vi "App - temperature sweep -- Pgg2.vi"() -> ()   [LabVIEW 2016]
uses:
  <vilib>/regexp/Match Regular Expression.xnode
  pair.ctl
  p9action control.ctl
  itc 503 box - control.ctl
  gas flow controller action.ctl
  ctl -- name dispatcher -- action.ctl
  countdown control.ctl
  NHMFL_Core/Libraries/Instruments/Temperature Controller/Controls/Set Point Aproach.ctl
  state.ctl
  save log.ctl
  resonant_ultrasound/Libraries/RUS/Controls/Sweep settings.ctl
  resonant_ultrasound/Libraries/RUS/Controls/Lock-in DAQ settings.ctl
  NHMFL_Core/Libraries/File/Controls/File formats.ctl
  NHMFL_Core/Libraries/File/Controls/Save data settings.ctl
  alarm clock control.ctl
  temperature indicator.ctl
  gas flow control - progress.ctl
  adaptive sweep UI controls.ctl
  next chunk -- algorithm.ctl
  Set Temperature PID - Control.ctl
  time in gamma mode control.ctl
  Sample_Temperature_Source_Control.ctl
  ITC Panel -- Hg.ctl
  gas flow controller control -- Pgg2.ctl
  resonant_ultrasound/Libraries/RUS/Controls/Lockin mode.ctl
  oxford ITC legacy-new - control.ctl
panel:
  in  "sweep folder path":path=path "C:/data/Ultrasound/birdcage/0_test"
  in  "Tab: everything":T1(tab) caption="Tab Control"
  in  "Tab: RUS controls":T2(tab)
  in  "RUS settings":enum32{"main", "save and staff"}(tab)
  in  "adaptive sweep settings":T3={"time gap (min) "=0.0, "Bypass error dialog"=TRUE, "range factor"=1.2, "min gamma(kHz)"=0.005, "max step(Hz)"=1500.0, "min step(Hz)"=0.001, "save freq units"=enum."kHz", "Zero signal?"=FALSE, "time in Gamma --OK"=FALSE, "scan mode"=enum."uniform", "power control mode "=enum."none", "time-in-gamma mode"=enum."uniform scan"}
  in  "Fast sweep settings":T6={"Update rate (Hz)"=200.0, "Start F, Hz"=2000000.0, "Stop F"=3000000.0, "Number of points"=5760, "Amplitude"=2.0, "Init&amplitude"=TRUE, "IF"=1000.0, "Time constant"=0.001} {"IF" format="%#_6p"; "Amplitude" min=0.0 max=2.5; "Number of points" format="%.0p"; "Stop F" format="%#_6p"; "Start F, Hz" format="%#_6p"; "Update rate (Hz)" format="%0.2f"}
  in  "Save data settings":T7={"Save data"=TRUE, "Data Root Path"=path "E:/Technique/RUS/Saphire/Saphire_piece1/1_test", "File Prefix"="291.30300K_2000_3000_2.00000V_0.00000T_Jul26-2016__14-58-15_", "File Format"=enum."BINARY", "Save column names"=FALSE, "File Comments"="\r\nColumns:Frequency\\tX\\tY\r\n    ITC Temp= 299.200000\r\n    LTC Temp= 0.000000\r\n          ITC_set=295.00000\r\n", "User/Prj"="<User Name/Project Description>"}
  in  "Lock-in DAQ settings":T9={"Lockin mode"=enum."Pitaya", "DAQmx Device"="", "SR Lockin"="GPIB0::10::INSTR", "Clock Multiplier"=64, "Low-pass filter"=enum."No filtering", "Ranges and couplings "=[{"Range"=2.5, "Coupling"=10106}], "Samples per read"=20, "Record IF"=FALSE, "Auto-phase"=FALSE, "RP IP Addres"="172.20.117.190"} {"Ranges and couplings"."Coupling" items=["default"=-1, "RSE"=10083, "NRSE"=10078, "Differential"=10106, "Pseudodifferential"=12529]}
  out "sweep time  (min)":dbl=1.05
  out "sweep time (sec)":i32=63
  out "kHz/second":dbl=31.746031746031747
  in  "RUS loop":bool
  in  "RUS zeroed":bool
  in  "read AH every # sec":dbl=1.7
  in  "plot":T11(ring)=enum."Capac vs Temp"
  out "temperature":dbl=198.969
  out "time(min)":dbl
  out "Capacitance":dbl=0.600435
  out "Loss":dbl=0.00206
  in  "save every # (min)":dbl=7.12
  in  "history length (min)":dbl=60.0
  in  "Sweep folder path":path=path "C:/data/RUS/Experiment/ProbeTest/cantilever/Hg1201-2-2/sweep1"
  in  "VISA - AH2500":refnum<visa-resource-name>="GPIB0::28::INSTR"
  in  "take cantilever reading":bool=TRUE
  out "Plot: capacitance":cluster{dbl[], dbl[]}[](graph)
  in  "plot lever  ?":bool
  in  "show plot pallets ?":bool
  in  "Tab: ITC controls":enum32{"display", "gas ", "progress"}(tab)
  in  "set Temperature target":T12(ring)=enum."set T -> ITC (oxford)"
  in  "Set Temperature PID":T13={"mode "=enum."bezier", "set temperature?"=FALSE, "Time(min)"=1492.1025, "Temperature(K)"=295.0, "OK?"=TRUE, "interval(sec)"=6.153}
  in  "ITC panel":T14={"in sweep"=FALSE, "start/stop sweep"=FALSE, "ITC state"="X0A1C2S01H1L0\r", "gas MANUAL"=TRUE, "gas AUTO"=FALSE, "local"=TRUE, "unlocked"=TRUE, "remote"=FALSE, "locked"=FALSE, "gas (%)"=0.0999, "heater AUTO"=FALSE, "heater MANUAL"=TRUE, "state indicator  (fake)"="NOT in sweep", "heater (V)"=0.0001, "Sweep"=FALSE}
  in  "itc box: set temperature to: value":dbl=295.0
  in  "set temperature to":bool
  in  "interaction with itc":T15(ring)
  in  "set heater to":bool
  in  "itc box: set heater to: value":dbl
  in  "itc box protocol selector":T16
  in  "gas flow controller":T17={"UP step (%)"=0.5, "ramp DOWN"=FALSE, "ramp UP"=FALSE, "idle"=TRUE, "UP time (min)"=20.0, "ramp step (%)"=0.1, "check (min)"=3.0, "DOWN step (%)"=0.5, "DOWN time (min)"=20.0, "to"=0.1, "last (min)"=1.6407999999999996, "below"=TRUE, "above"=FALSE, "Control Gas"=FALSE, "upper"=7.0, "lower"=3.0, "heater"=0.00010000000000000003, "in range"=FALSE, "gas, %"=0.0999, "ramp Up progress"={"(total # of ramp steps)"=5, "ramp time step (sec)"=240, "steps so far"=0, "state"=enum."normal"}, "ramp Down progress"={"(total # of ramp steps)"=5, "ramp time step (sec)"=240, "steps so far"=0, "state"=enum."normal"}, "state"=enum."normal", "set gas"=FALSE}
  out "ramp Down progress":T18={"(total # of ramp steps)"=5, "ramp time step (sec)"=240, "steps so far"=0, "state"=enum."normal"}
  out "ramp Up progress":T18={"(total # of ramp steps)"=5, "ramp time step (sec)"=240, "steps so far"=0, "state"=enum."normal"}
  in  "Tab: plots":enum32{"Plot:  gas/heater", "Plot: temperayre"}(tab)=enum."Plot: temperayre"
  out "Plot: heater/gas":cluster{dbl[], dbl[]}[](graph)
  out "Plot: temperature":cluster{dbl[], dbl[]}[](graph)=[{array[586 elements], [0.0, 0.0, 0.0, 0.0, 0.0, 0.0, 0.0, 0.0, 0.0, 0.0, 0.0, 0.0, 0.0, 0.0, 0.0, 0.0, 0.0, 0.0, 0.0, 0.0, 0.0, 0.0, 0.0, 0.0, 0.0, 0.0, 0.0, 0.0, 0.0, 0.0, 0.0, 0.0, 0.0, 0.0, 0.0, 0.0, 0.0, 0.0, 0.0, 0.0, 0.0, 0.0, 0.0, 0.0, 0.0, 0.0, 0.0, 0.0, 0.0, 0.0, 0.0, 0.0, 0.0, 0.0, 0.0, 0.0, 0.0, 0.0, 0.0, 0.0, 0.0, 0.0, 0.0, 0.0, 0.0, 0.0, 0.0, 0.0, 0.0, 0.0, 0.0, 0.0, 0.0, 0.0, 0.0, 0.0, 0.0, 0.0, 0.0, 0.0, 0.0, 0.0, 0.0, 0.0, 0.0, 0.0, 0.0, 0.0, 0.0, 0.0, 0.0, 0.0, 0.0, 0.0, 0.0, 0.0, 0.0, 0.0, 0.0, 0.0, 0.0, 0.0, 0.0, 0.0, 0.0, 0.0, 0.0, 0.0, 0.0, 0.0, 0.0, 0.0, 0.0, 0.0, 0.0, 0.0, 0.0, 0.0, 0.0, 0.0, 0.0, 0.0, 0.0, 0.0, 0.0, 0.0, 0.0, 0.0, 0.0, 0.0, 0.0, 0.0, 0.0, 0.0, 0.0, 0.0, 0.0, 0.0, 0.0, 0.0, 0.0, 0.0, 0.0, 0.0, 0.0, 0.0, 0.0, 0.0, 0.0, 0.0, 0.0, 0.0, 0.0, 0.0, 0.0, 0.0, 0.0, 0.0, 0.0, 0.0, 0.0, 0.0, 0.0, 0.0, 0.0, 0.0, 0.0, 0.0, 0.0, 0.0, 0.0, 0.0, 0.0, 0.0, 0.0, 0.0, 0.0, 0.0, 0.0, 0.0, 0.0, 0.0, 0.0, 0.0, 0.0, 0.0, 0.0, 0.0, 0.0, 0.0, 0.0, 0.0, 0.0, 0.0, 0.0, 0.0, 0.0, 0.0, 0.0, 0.0, 0.0, 0.0, 0.0, 0.0, 0.0, 0.0, 0.0, 0.0, 0.0, 0.0, 0.0, 0.0, 0.0, 0.0, 0.0, 0.0, 0.0, 0.0, 0.0, 0.0, 0.0, 0.0, 0.0, 0.0, 0.0, 0.0, 0.0, 0.0, 0.0, 0.0, 0.0, 0.0, 0.0, 0.0, 0.0, 0.0, 0.0, 0.0, 0.0, 0.0, 0.0, 0.0, 0.0, 0.0, 0.0, 0.0, 0.0, 0.0, 0.0, 0.0, 0.0, 0.0, 0.0, 0.0, 0.0, 0.0, 0.0, 0.0, 0.0, 0.0, 0.0, 0.0, 0.0, 0.0, 0.0, 0.0, 0.0, 0.0, 0.0, 0.0, 0.0, 0.0, 0.0, 0.0, 0.0, 0.0, 0.0, 0.0, 0.0, 0.0, 0.0, 0.0, 0.0, 0.0, 0.0, 0.0, 0.0, 0.0, 0.0, 0.0, 0.0, 0.0, 0.0, 0.0, 0.0, 0.0, 0.0, 0.0, 0.0, 0.0, 0.0, 0.0, 0.0, 0.0, 0.0, 0.0, 0.0, 0.0, 0.0, 0.0, 0.0, 0.0, 0.0, 0.0, 0.0, 0.0, 0.0, 0.0, 0.0, 0.0, 0.0, 0.0, 0.0, 0.0, 0.0, 0.0, 0.0, 0.0, 0.0, 0.0, 0.0, 0.0, 0.0, 0.0, 0.0, 0.0, 0.0, 0.0, 0.0, 0.0, 0.0, 0.0, 0.0, 0.0, 0.0, 0.0, 0.0, 0.0, 0.0, 0.0, 0.0, 0.0, 0.0, 0.0, 0.0, 0.0, 0.0, 0.0, 0.0, 0.0, 0.0, 0.0, 0.0, 0.0, 0.0, 0.0, 0.0, 0.0, 0.0, 0.0, 0.0, 0.0, 0.0, 0.0, 0.0, 0.0, 0.0, 0.0, 0.0, 0.0, 0.0, 0.0, 0.0, 0.0, 0.0, 0.0, 0.0, 0.0, 0.0, 0.0, 0.0, 0.0, 0.0, 0.0, 0.0, 0.0, 0.0, 0.0, 0.0, 0.0, 0.0, 0.0, 0.0, 0.0, 0.0, 0.0, 0.0, 0.0, 0.0, 0.0, 0.0, 0.0, 0.0, 0.0, 0.0, 0.0, 0.0, 0.0, 0.0, 0.0, 0.0, 0.0, 0.0, 0.0, 0.0, 0.0, 0.0, 0.0, 0.0, 0.0, 0.0, 0.0, 0.0, 0.0, 0.0, 0.0, 0.0, 0.0, 0.0, 0.0, 0.0, 0.0, 0.0, 0.0, 0.0, 0.0, 0.0, 0.0, 0.0, 0.0, 0.0, 0.0, 0.0, 0.0, 0.0, 0.0, 0.0, 0.0, 0.0, 0.0, 0.0, 0.0, 0.0, 0.0, 0.0, 0.0, 0.0, 0.0, 0.0, 0.0, 0.0, 0.0, 0.0, 0.0, 0.0, 0.0, 0.0, 0.0, 0.0, 0.0, 0.0, 0.0, 0.0, 0.0, 0.0, 0.0, 0.0, 0.0, 0.0, 0.0, 0.0, 0.0, 0.0, 0.0, 0.0, 0.0, 0.0, 0.0, 0.0, 0.0, 0.0, 0.0, 0.0, 0.0, 0.0, 0.0, 0.0, 0.0, 0.0, 0.0, 0.0, 0.0, 0.0, 0.0, 0.0, 0.0, 0.0, 0.0, 0.0, 0.0, 0.0, 0.0, 0.0, 0.0, 0.0, 0.0, 0.0, 0.0, 0.0, 0.0, 0.0, 0.0, 0.0, 0.0, 0.0, 0.0, 0.0, 0.0, 0.0, 295.0, 295.0, 295.0, 295.0, 295.0, 295.0, 295.0, 295.0, 295.0, 295.0, 295.0, 295.0, 295.0, 295.0, 295.0, 295.0, 295.0, 295.0, 295.0, 295.0, 295.0, 295.0, 295.0, 295.0, 295.0, 295.0, 295.0, 295.0, 295.0, 295.0, 295.0, 295.0, 295.0, 295.0, 295.0, 295.0, 295.0, 295.0, 295.0, 295.0, 295.0, 295.0, 295.0, 295.0, 295.0, 295.0, 295.0]}, {array[586 elements], [0.0, 0.0, 0.0, 0.0, 0.0, 0.0, 0.0, 0.0, 0.0, 0.0, 0.0, 0.0, 0.0, 0.0, 0.0, 0.0, 0.0, 0.0, 0.0, 0.0, 0.0, 0.0, 0.0, 0.0, 0.0, 0.0, 0.0, 0.0, 0.0, 0.0, 0.0, 0.0, 0.0, 0.0, 0.0, 0.0, 0.0, 0.0, 0.0, 0.0, 0.0, 0.0, 0.0, 0.0, 0.0, 0.0, 0.0, 0.0, 0.0, 0.0, 0.0, 0.0, 0.0, 0.0, 0.0, 0.0, 0.0, 0.0, 0.0, 0.0, 0.0, 0.0, 0.0, 0.0, 0.0, 0.0, 0.0, 0.0, 0.0, 0.0, 0.0, 0.0, 0.0, 0.0, 0.0, 0.0, 0.0, 0.0, 0.0, 0.0, 0.0, 0.0, 0.0, 0.0, 0.0, 0.0, 0.0, 0.0, 0.0, 0.0, 0.0, 0.0, 0.0, 0.0, 0.0, 0.0, 0.0, 0.0, 0.0, 0.0, 0.0, 0.0, 0.0, 0.0, 0.0, 0.0, 0.0, 0.0, 0.0, 0.0, 0.0, 0.0, 0.0, 0.0, 0.0, 0.0, 0.0, 0.0, 0.0, 0.0, 0.0, 0.0, 0.0, 0.0, 0.0, 0.0, 0.0, 0.0, 0.0, 0.0, 0.0, 0.0, 0.0, 0.0, 0.0, 0.0, 0.0, 0.0, 0.0, 0.0, 0.0, 0.0, 0.0, 0.0, 0.0, 0.0, 0.0, 0.0, 0.0, 0.0, 0.0, 0.0, 0.0, 0.0, 0.0, 0.0, 0.0, 0.0, 0.0, 0.0, 0.0, 0.0, 0.0, 0.0, 0.0, 0.0, 0.0, 0.0, 0.0, 0.0, 0.0, 0.0, 0.0, 0.0, 0.0, 0.0, 0.0, 0.0, 0.0, 0.0, 0.0, 0.0, 0.0, 0.0, 0.0, 0.0, 0.0, 0.0, 0.0, 0.0, 0.0, 0.0, 0.0, 0.0, 0.0, 0.0, 0.0, 0.0, 0.0, 0.0, 0.0, 0.0, 0.0, 0.0, 0.0, 0.0, 0.0, 0.0, 0.0, 0.0, 0.0, 0.0, 0.0, 0.0, 0.0, 0.0, 0.0, 0.0, 0.0, 0.0, 0.0, 0.0, 0.0, 0.0, 0.0, 0.0, 0.0, 0.0, 0.0, 0.0, 0.0, 0.0, 0.0, 0.0, 0.0, 0.0, 0.0, 0.0, 0.0, 0.0, 0.0, 0.0, 0.0, 0.0, 0.0, 0.0, 0.0, 0.0, 0.0, 0.0, 0.0, 0.0, 0.0, 0.0, 0.0, 0.0, 0.0, 0.0, 0.0, 0.0, 0.0, 0.0, 0.0, 0.0, 0.0, 0.0, 0.0, 0.0, 0.0, 0.0, 0.0, 0.0, 0.0, 0.0, 0.0, 0.0, 0.0, 0.0, 0.0, 0.0, 0.0, 0.0, 0.0, 0.0, 0.0, 0.0, 0.0, 0.0, 0.0, 0.0, 0.0, 0.0, 0.0, 0.0, 0.0, 0.0, 0.0, 0.0, 0.0, 0.0, 0.0, 0.0, 0.0, 0.0, 0.0, 0.0, 0.0, 0.0, 0.0, 0.0, 0.0, 0.0, 0.0, 0.0, 0.0, 0.0, 0.0, 0.0, 0.0, 0.0, 0.0, 0.0, 0.0, 0.0, 0.0, 0.0, 0.0, 0.0, 0.0, 0.0, 0.0, 0.0, 0.0, 0.0, 0.0, 0.0, 0.0, 0.0, 0.0, 0.0, 0.0, 0.0, 0.0, 0.0, 0.0, 0.0, 0.0, 0.0, 0.0, 0.0, 0.0, 0.0, 0.0, 0.0, 0.0, 0.0, 0.0, 0.0, 0.0, 0.0, 0.0, 0.0, 0.0, 0.0, 0.0, 0.0, 0.0, 0.0, 0.0, 0.0, 0.0, 0.0, 0.0, 0.0, 0.0, 0.0, 0.0, 0.0, 0.0, 0.0, 0.0, 0.0, 0.0, 0.0, 0.0, 0.0, 0.0, 0.0, 0.0, 0.0, 0.0, 0.0, 0.0, 0.0, 0.0, 0.0, 0.0, 0.0, 0.0, 0.0, 0.0, 0.0, 0.0, 0.0, 0.0, 0.0, 0.0, 0.0, 0.0, 0.0, 0.0, 0.0, 0.0, 0.0, 0.0, 0.0, 0.0, 0.0, 0.0, 0.0, 0.0, 0.0, 0.0, 0.0, 0.0, 0.0, 0.0, 0.0, 0.0, 0.0, 0.0, 0.0, 0.0, 0.0, 0.0, 0.0, 0.0, 0.0, 0.0, 0.0, 0.0, 0.0, 0.0, 0.0, 0.0, 0.0, 0.0, 0.0, 0.0, 0.0, 0.0, 0.0, 0.0, 0.0, 0.0, 0.0, 0.0, 0.0, 0.0, 0.0, 0.0, 0.0, 0.0, 0.0, 0.0, 0.0, 0.0, 0.0, 0.0, 0.0, 0.0, 0.0, 0.0, 0.0, 0.0, 0.0, 0.0, 0.0, 0.0, 0.0, 0.0, 0.0, 0.0, 0.0, 0.0, 0.0, 0.0, 0.0, 0.0, 0.0, 0.0, 0.0, 0.0, 0.0, 0.0, 0.0, 0.0, 0.0, 0.0, 0.0, 0.0, 0.0, 0.0, 0.0, 0.0, 0.0, 0.0, 0.0, 0.0, 0.0, 0.0, 0.0, 0.0, 0.0, 0.0, 0.0, 0.0, 0.0, 0.0, 0.0, 0.0, 0.0, 0.0, 0.0, 0.0, 0.0, 0.0, 0.0, 0.0, 0.0, 0.0, 0.0, 0.0, 0.0, 0.0, 0.0, 0.0, 0.0, 0.0, 299.8818, 299.8725, 299.8681, 299.8587, 299.8481, 299.8385, 299.8337, 299.8248, 299.8151, 299.8057, 299.7963, 299.7864, 299.7782, 299.7712, 299.7639, 299.7545, 299.7469, 299.7379, 299.7298, 299.7206, 299.7145, 299.7075, 299.6935, 299.6904, 299.681, 299.6731, 299.6655, 299.639, 299.6394, 299.6394, 299.6338, 299.6278, 299.6215, 299.6071, 299.6045, 299.5932, 299.5878, 299.5787, 299.5757, 299.5664, 299.5592, 299.551, 299.5432, 299.5356, 299.5272, 299.5242, 299.5086]}, {array[586 elements], [0.0, 0.0, 0.0, 0.0, 0.0, 0.0, 0.0, 0.0, 0.0, 0.0, 0.0, 0.0, 0.0, 0.0, 0.0, 0.0, 0.0, 0.0, 0.0, 0.0, 0.0, 0.0, 0.0, 0.0, 0.0, 0.0, 0.0, 0.0, 0.0, 0.0, 0.0, 0.0, 0.0, 0.0, 0.0, 0.0, 0.0, 0.0, 0.0, 0.0, 0.0, 0.0, 0.0, 0.0, 0.0, 0.0, 0.0, 0.0, 0.0, 0.0, 0.0, 0.0, 0.0, 0.0, 0.0, 0.0, 0.0, 0.0, 0.0, 0.0, 0.0, 0.0, 0.0, 0.0, 0.0, 0.0, 0.0, 0.0, 0.0, 0.0, 0.0, 0.0, 0.0, 0.0, 0.0, 0.0, 0.0, 0.0, 0.0, 0.0, 0.0, 0.0, 0.0, 0.0, 0.0, 0.0, 0.0, 0.0, 0.0, 0.0, 0.0, 0.0, 0.0, 0.0, 0.0, 0.0, 0.0, 0.0, 0.0, 0.0, 0.0, 0.0, 0.0, 0.0, 0.0, 0.0, 0.0, 0.0, 0.0, 0.0, 0.0, 0.0, 0.0, 0.0, 0.0, 0.0, 0.0, 0.0, 0.0, 0.0, 0.0, 0.0, 0.0, 0.0, 0.0, 0.0, 0.0, 0.0, 0.0, 0.0, 0.0, 0.0, 0.0, 0.0, 0.0, 0.0, 0.0, 0.0, 0.0, 0.0, 0.0, 0.0, 0.0, 0.0, 0.0, 0.0, 0.0, 0.0, 0.0, 0.0, 0.0, 0.0, 0.0, 0.0, 0.0, 0.0, 0.0, 0.0, 0.0, 0.0, 0.0, 0.0, 0.0, 0.0, 0.0, 0.0, 0.0, 0.0, 0.0, 0.0, 0.0, 0.0, 0.0, 0.0, 0.0, 0.0, 0.0, 0.0, 0.0, 0.0, 0.0, 0.0, 0.0, 0.0, 0.0, 0.0, 0.0, 0.0, 0.0, 0.0, 0.0, 0.0, 0.0, 0.0, 0.0, 0.0, 0.0, 0.0, 0.0, 0.0, 0.0, 0.0, 0.0, 0.0, 0.0, 0.0, 0.0, 0.0, 0.0, 0.0, 0.0, 0.0, 0.0, 0.0, 0.0, 0.0, 0.0, 0.0, 0.0, 0.0, 0.0, 0.0, 0.0, 0.0, 0.0, 0.0, 0.0, 0.0, 0.0, 0.0, 0.0, 0.0, 0.0, 0.0, 0.0, 0.0, 0.0, 0.0, 0.0, 0.0, 0.0, 0.0, 0.0, 0.0, 0.0, 0.0, 0.0, 0.0, 0.0, 0.0, 0.0, 0.0, 0.0, 0.0, 0.0, 0.0, 0.0, 0.0, 0.0, 0.0, 0.0, 0.0, 0.0, 0.0, 0.0, 0.0, 0.0, 0.0, 0.0, 0.0, 0.0, 0.0, 0.0, 0.0, 0.0, 0.0, 0.0, 0.0, 0.0, 0.0, 0.0, 0.0, 0.0, 0.0, 0.0, 0.0, 0.0, 0.0, 0.0, 0.0, 0.0, 0.0, 0.0, 0.0, 0.0, 0.0, 0.0, 0.0, 0.0, 0.0, 0.0, 0.0, 0.0, 0.0, 0.0, 0.0, 0.0, 0.0, 0.0, 0.0, 0.0, 0.0, 0.0, 0.0, 0.0, 0.0, 0.0, 0.0, 0.0, 0.0, 0.0, 0.0, 0.0, 0.0, 0.0, 0.0, 0.0, 0.0, 0.0, 0.0, 0.0, 0.0, 0.0, 0.0, 0.0, 0.0, 0.0, 0.0, 0.0, 0.0, 0.0, 0.0, 0.0, 0.0, 0.0, 0.0, 0.0, 0.0, 0.0, 0.0, 0.0, 0.0, 0.0, 0.0, 0.0, 0.0, 0.0, 0.0, 0.0, 0.0, 0.0, 0.0, 0.0, 0.0, 0.0, 0.0, 0.0, 0.0, 0.0, 0.0, 0.0, 0.0, 0.0, 0.0, 0.0, 0.0, 0.0, 0.0, 0.0, 0.0, 0.0, 0.0, 0.0, 0.0, 0.0, 0.0, 0.0, 0.0, 0.0, 0.0, 0.0, 0.0, 0.0, 0.0, 0.0, 0.0, 0.0, 0.0, 0.0, 0.0, 0.0, 0.0, 0.0, 0.0, 0.0, 0.0, 0.0, 0.0, 0.0, 0.0, 0.0, 0.0, 0.0, 0.0, 0.0, 0.0, 0.0, 0.0, 0.0, 0.0, 0.0, 0.0, 0.0, 0.0, 0.0, 0.0, 0.0, 0.0, 0.0, 0.0, 0.0, 0.0, 0.0, 0.0, 0.0, 0.0, 0.0, 0.0, 0.0, 0.0, 0.0, 0.0, 0.0, 0.0, 0.0, 0.0, 0.0, 0.0, 0.0, 0.0, 0.0, 0.0, 0.0, 0.0, 0.0, 0.0, 0.0, 0.0, 0.0, 0.0, 0.0, 0.0, 0.0, 0.0, 0.0, 0.0, 0.0, 0.0, 0.0, 0.0, 0.0, 0.0, 0.0, 0.0, 0.0, 0.0, 0.0, 0.0, 0.0, 0.0, 0.0, 0.0, 0.0, 0.0, 0.0, 0.0, 0.0, 0.0, 0.0, 0.0, 0.0, 0.0, 0.0, 0.0, 0.0, 0.0, 0.0, 0.0, 0.0, 0.0, 0.0, 0.0, 0.0, 0.0, 0.0, 0.0, 0.0, 0.0, 0.0, 0.0, 0.0, 0.0, 0.0, 0.0, 0.0, 0.0, 0.0, 0.0, 0.0, 0.0, 0.0, 0.0, 0.0, 0.0, 0.0, 0.0, 0.0, 0.0, 0.0, 0.0, 0.0, 0.0, 0.0, 0.0, 0.0, 0.0, 0.0, 0.0, 0.0, 291.442, 291.424, 291.446, 291.442, 291.414, 291.425, 291.433, 291.42, 291.41, 291.408, 291.414, 291.426, 291.417, 291.411, 291.407, 291.401, 291.407, 291.409, 291.388, 291.358, 291.355, 291.356, 291.349, 291.341, 291.315, 291.309, 291.316, 291.307, 291.299, 291.3, 291.307, 291.319, 291.313, 291.307, 291.313, 291.315, 291.317, 291.32, 291.33, 291.317, 291.316, 291.314, 291.317, 291.315, 291.303, 291.275, 291.282]}]
  in  "Tab: controls":enum32{"indicators", "counter", "boxes"}(tab)=enum."boxes"
  in  "temperature indicator panel":T19={"LTC T"=291.282, "ITC T"=299.5086, "ITC Set T"=295.0, "LTC T slope, K/min"=-0.03488517367717843, "heater i-average, V"=0.00010000000000000005, "heater slope, V/min"=2.130840846245559e-20, "LTC T i-average, K"=291.2722044403331, "ITC T i-average, K"=-0.008056232654941152, "gas"=0.0} {"ITC Set T" format="%.3g"; "ITC T" format="%.3g"; "LTC T" format="%.3g"; "gas" format="%.3g"; "ITC T i-average, K" format="%#.5f"; "LTC T i-average, K" format="%#.5f"; "heater i-average, V" format="%.3g"; "heater slope, V/min" format="%#.5f"; "LTC T slope, K/min" format="%#.5f"}
  in  "Tab : everything to zero":enum32{"Page 1", "Page 2"}(tab)
  in  "alarm":T20={"counter (min)"=0.0, "alarm"=FALSE, "start"=FALSE, "set (min)"=1600.0, "stop"=FALSE} {"set (min)" format="%_4f"; "counter (min)" format="%_4f"}
  in  "Tab : Overheat":enum32{"Page 1"}(tab)
  in  "Over heat Temperature":dbl=315.0
  in  "Overheat protection":bool
  in  "Overheat !!":bool
  in  "temperature boxes":T21={"LTC21 Address"="GPIB0::15::INSTR", "ITC503 Address"="GPIB0::24::INSTR", "ITC temperature"=299.5086, "ITC set temperature"=295.0, "LTC temperature"=291.282, "heater"=0.0001, "gas flow"=0.0999, "P"=9.3041, "D"=0.1, "I"=0.5885, "ITC state"="X0A0C2S00H0L0", "nonzero temperature"=291.282, "Field (T)"=0.0, "LakeShore340"="LPT1", "LS340 Adress"=11, "Sample Temperature Source"=enum."read T <- Neocera", "Neocera sensor"=1, "Magnetic Field Source"=enum."None", "field scale"=0.6578903516080653} {"field scale" format="%#_16g"}
  in  "plot?":bool=TRUE
  in  "PID timer":dbl(slide)=81.80999999993946 min=-28454336.0 max=2135380277.0 step=0.010000000000000002 scale=0.0..100.0 scale format="%#3_3f"
  out "PID OK":bool=TRUE
  out "PID":dbl[](array[numeric])=[9.304073011801927, 0.5884549840916852, 0.09999999999999996]
  out "PID temperature":dbl=299.6215
  out "Uploading ...":bool
  in  "Tab : Upload Sweep table":enum32{"Page 1"}(tab)
  out "Sweep Rates , min/K":dbl[](array[numeric])=[12.0, -0.0, 0.0, 0.0, 0.0, 0.0, 0.0, 0.0, 0.0, 0.0, 0.0, 0.0, 0.0, 0.0, 0.0, 0.0]
  out "current set temperature":dbl=50.0
  in  "set temperature":dbl=295.0
  in  "new sweep table":dbl[][](array[numeric])=[[200.0, 1000.0, 0.0], [100.0, 500.0, 0.0], [0.0, 0.0, 0.0], [0.0, 0.0, 0.0], [0.0, 0.0, 0.0], [0.0, 0.0, 0.0], [0.0, 0.0, 0.0], [0.0, 0.0, 0.0], [0.0, 0.0, 0.0], [0.0, 0.0, 0.0], [0.0, 0.0, 0.0], [0.0, 0.0, 0.0], [0.0, 0.0, 0.0], [0.0, 0.0, 0.0], [0.0, 0.0, 0.0], [70.0, 0.0, 0.0]]
  in  "Read Sweep Table in the box":bool
  out "Sweep Table":dbl[][](array[numeric])=[[70.0, 240.0, 1000.0], [0.0, 0.0, 0.0], [0.0, 0.0, 0.0], [0.0, 0.0, 0.0], [0.0, 0.0, 0.0], [0.0, 0.0, 0.0], [0.0, 0.0, 0.0], [0.0, 0.0, 0.0], [0.0, 0.0, 0.0], [0.0, 0.0, 0.0], [0.0, 0.0, 0.0], [0.0, 0.0, 0.0], [0.0, 0.0, 0.0], [0.0, 0.0, 0.0], [0.0, 0.0, 0.0], [70.0, 0.0, 0.0]]
  in  "upload new sweep table":bool
  out "index":dbl[][](array[numeric])=[[0.0, 1200.0, 0.0], [1.0, 1200.0, 0.0], [2.0, 500.0, 0.0], [3.0, 1399.0, 0.0], [4.0, 10.0, 1399.0], [5.0, 10.0, 1399.0], [6.0, 0.0, 0.0], [7.0, 0.0, 0.0], [8.0, 0.0, 0.0], [9.0, 0.0, 0.0], [10.0, 0.0, 0.0], [11.0, 0.0, 0.0], [12.0, 0.0, 0.0], [13.0, 0.0, 0.0], [14.0, 0.0, 0.0], [15.0, 0.0, 0.0]]
  out "date string Array":string[](array[string])=["Fri, Mar 07, 2014   :   11:06 AM", "Fri, Mar 07, 2014   :   3:06 PM"]
  in  "Rates , min/K":dbl[](array[numeric])=[12.0, -0.0, 0.0, 0.0, 0.0, 0.0, 0.0, 0.0, 0.0, 0.0, 0.0, 0.0, 0.0, 0.0, 0.0, 0.0]
  in  "use":bool
  out "writing log to":string="E:\\data\\Ultrasound\\Experiment\\ProbeTest\\Birdcage\\saphire-test\\1_test\\itc_log\\Stability_101113.dat"
  out "log line":string="time=Oct11,2013__13:45:08\tLTC=0.00000\tITC=0.00000\t ITC_set=0.00000\t\t filename=300.00000K_200_1000_2.10000V_0.00000T_Oct11-2013__13-45-08_101113.dat\t"
  out "saving log to":string
  out "saving sweep table to":string
  in  "save log":T23={"file path"=path "E:/data/Ultrasound/Experiment/ProbeTest/Birdcage/saphire-test/1_test", "Save log?"=TRUE, "every # of sec"=64}
  in  "set gas % to":dbl=10.0
  out "9ctl OK":bool=TRUE
  out "minutes":dbl=4.717316666666666
  out "milliseconds per cycle":u32=6153
  out "seconds per cycle":dbl=6.153
  out "file name prefix":string="291.30300K_2000_3000_2.00000V_0.00000T_Jul26-2016__14-58-15_"
  out "x-y":dbl=30.765000000000015
  out "seconds":dbl=283.039
  in  "error in":errorcluster
  # "the paths are copied from \"data root path\" in the first page"
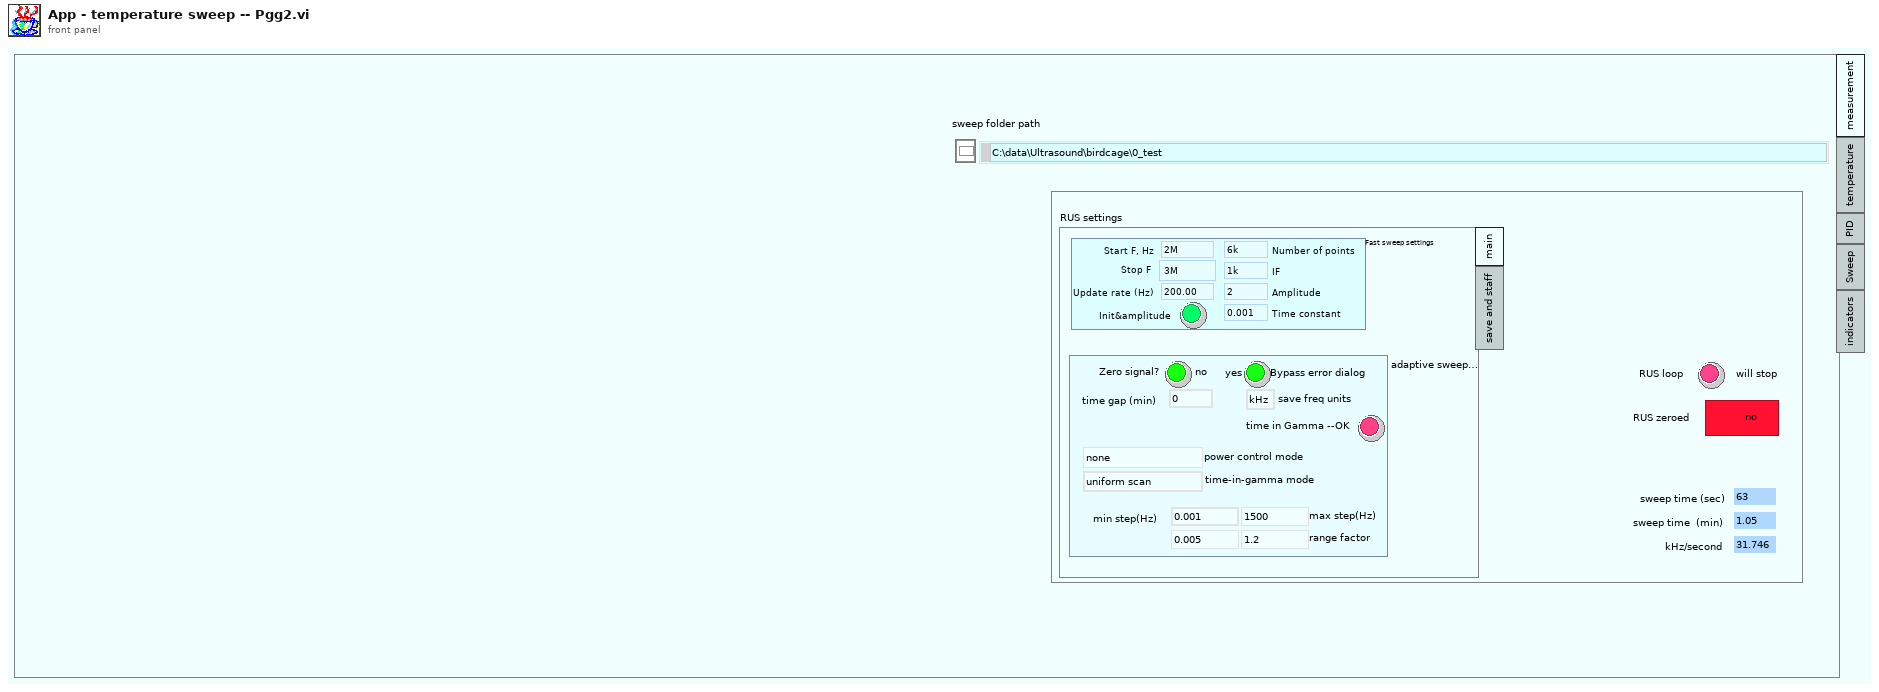
[diagram p1: front panel]
types:
  T1 = enum32{"measurement", "temperature", "PID", "Sweep", "indicators"}
  T2 = enum32{"Resonant Ultrasound", "Cantilever", "Strain"}
  T3 = typedef "adaptive sweep UI controls.ctl" = cluster{"time gap (min) ":dbl, "Bypass error dialog":bool, "range factor":dbl, "min gamma(kHz)":dbl, "max step(Hz)":dbl, "min step(Hz)":dbl, "save freq units":enum16{"kHz", "Hz"}, "Zero signal?":bool, "time in Gamma --OK":bool, "scan mode":T4, "power control mode ":enum16{"power vs Temp", "power vs Time", "none"}, "time-in-gamma mode":T5}
  T4 = typedef "next chunk -- algorithm.ctl" = enum16{"peak position is known", "uniform", "predictive"}
  T5 = typedef "time in gamma mode control.ctl" = enum16{"same for all", "each one different", "uniform scan"}
  T6 = typedef "Sweep settings.ctl" = cluster{"Update rate (Hz)":dbl, "Start F, Hz":dbl, "Stop F":dbl, "Number of points":i32, "Amplitude":dbl, "Init&amplitude":bool, "IF":dbl, "Time constant":dbl}
  T7 = typedef "Save data settings.ctl" = cluster{"Save data":bool, "Data Root Path":path, "File Prefix":string, "File Format":T8, "Save column names":bool, "File Comments":string, "User/Prj":string}
  T8 = typedef "File formats.ctl" = enum16{"TDMS", "ASCII", "BINARY"}
  T9 = typedef "Lock-in DAQ settings.ctl" = cluster{"Lockin mode":T10, "DAQmx Device":tag, "SR Lockin":refnum<visa-resource-name>, "Clock Multiplier":i32, "Low-pass filter":enum16{"No filtering", "Butterworth", "Bessel"}, "Ranges and couplings ":cluster{"Range":dbl, "Coupling":i32}[], "Samples per read":i32, "Record IF":bool, "Auto-phase":bool, "RP IP Addres":string}
  T10 = typedef "Lockin mode.ctl" = enum16{"SRS", "NI-DAQ", "Pitaya"}
  T11 = enum16{"Capac vs Time", "Capac vs Temp", "Loss  vs Time", "Loss vs Temp", "Delta Cap vs Temp"}
  T12 = enum16{"set T -> LTC (neocera)", "set T -> ITC (oxford)"}
  T13 = typedef "Set Temperature PID - Control.ctl" = cluster{"mode ":enum16{"bezier", "sine wave"}, "set temperature?":bool, "Time(min)":dbl, "Temperature(K)":dbl, "OK?":bool, "interval(sec)":dbl}
  T14 = typedef "ITC Panel -- Hg.ctl" = cluster{"in sweep":bool, "start/stop sweep":bool, "ITC state":string, "gas MANUAL":bool, "gas AUTO":bool, "local":bool, "unlocked":bool, "remote":bool, "locked":bool, "gas (%)":dbl, "heater AUTO":bool, "heater MANUAL":bool, "state indicator  (fake)":string, "heater (V)":dbl, "Sweep":bool}
  T15 = enum16{"use oxford ITC", "do not use oxford ITC"}
  T16 = typedef "oxford ITC legacy-new - control.ctl" = enum16{"legacy", "new"}
  T17 = typedef "gas flow controller control -- Pgg2.ctl" = cluster{"UP step (%)":dbl, "ramp DOWN":bool, "ramp UP":bool, "idle":bool, "UP time (min)":dbl, "ramp step (%)":dbl, "check (min)":dbl, "DOWN step (%)":dbl, "DOWN time (min)":dbl, "to":dbl, "last (min)":dbl, "below":bool, "above":bool, "Control Gas":bool, "upper":dbl, "lower":dbl, "heater":dbl, "in range":bool, "gas, %":dbl, "ramp Up progress":T18, "ramp Down progress":T18, "state":enum16{"normal", "ramp up", "ramp down"}, "set gas":bool}
  T18 = typedef "gas flow control - progress.ctl" = cluster{"(total # of ramp steps)":i32, "ramp time step (sec)":i32, "steps so far":i32, "state":enum16{"normal", "ramp up", "ramp down"}}
  T19 = typedef "temperature indicator.ctl" = cluster{"LTC T":dbl, "ITC T":dbl, "ITC Set T":dbl, "LTC T slope, K/min":dbl, "heater i-average, V":dbl, "heater slope, V/min":dbl, "LTC T i-average, K":dbl, "ITC T i-average, K":dbl, "gas":dbl}
  T20 = typedef "alarm clock control.ctl" = cluster{"counter (min)":dbl, "alarm":bool, "start":bool, "set (min)":dbl, "stop":bool}
  T21 = typedef "state.ctl" = cluster{"LTC21 Address":refnum<visa-resource-name>, "ITC503 Address":refnum<visa-resource-name>, "ITC temperature":dbl, "ITC set temperature":dbl, "LTC temperature":dbl, "heater":dbl, "gas flow":dbl, "P":dbl, "D":dbl, "I":dbl, "ITC state":string, "nonzero temperature":dbl, "Field (T)":dbl, "LakeShore340":refnum<visa-resource-name>, "LS340 Adress":i16, "Sample Temperature Source":T22, "Neocera sensor":i32, "Magnetic Field Source":enum16{"None", "20T", "DTM"}, "field scale":dbl}
  T22 = typedef "Sample_Temperature_Source_Control.ctl" = enum16{"read T <- LakeShore 340", "read T <- Neocera"}
  T23 = typedef "save log.ctl" = cluster{"file path":path, "Save log?":bool, "every # of sec":i32}
  T24 = typedef "pair.ctl" = cluster{"num":i32, "bool":bool, "string":string}
  T25 = typedef "ctl -- name dispatcher -- action.ctl" = enum16{"peak frequency", "peak frequency DUMP", "peak gamma DUMP", "peak gamma", "peak frequency TEST", "peak gamma TEST", "ultrasonic power", "time in gamma", "set temperature ", "set temperature timer", "peak default gamma", "last scan file", "peak freq gamma TEST", "peak NAMES", "errors", "P_I_D", "P", "I", "D", "power vs time", "power vs time TIMER", "void", "power log", "set temperature - SINE", "itc ltc log", "peak - time in gamma"}
  T26 = typedef "file -- scan filename.ctl" = cluster{"mmddyy (str)":string, "counter (str)":string, "to F (kHz)":dbl, "from F (kHz)":dbl, "temperature (K)":dbl, "date/time string":string, "time stamp":timestamp, "base name":string, "temperature (str)":string, "from F (str)":string, "to F (str)":string, "format":enum16{"no date string", "with date string"}, "power (V)":dbl, "power (str) ":string, "Magn Field (T)":dbl, "Magn Field (str)":string}
  T27 = cluster{"temperature array":dbl[], "delta capacitance array":dbl[]}
  T28 = cluster{"temperature array":dbl[], "delta capacitance array":dbl[]}[]
  T29 = typedef "p9action control.ctl" = enum16{"init", "check", "reset", "log", "message", "change path"}
  T30 = typedef "countdown control.ctl" = enum16{"check", "start", "reset cont", "stop", "reset once"}
  T31 = typedef "gas flow controller action.ctl" = enum16{"check", "force UP", "stop UP/DOWN", "force DOWN", "init", "set gas to", "turn off", "turn on", "idle", "update parameters", "parse", "set gas"}
  T32 = typedef "itc 503 box - control.ctl" = enum16{"heater manual and zero", "heater auto", "upload D", "upload I", "upload P", "shut off", "init", "read sweep table", "disable", "enable", "read state", "set gas to", "stop sweep", "start sweep", "test", "set temperature to", "write sweep table", "-void", "set heater to"}
  T33 = enum16{"table to rates", "rates to table", "other"}
  T34 = enum16{"parse", "start sweep", "stop sweep", "heater auto", "heater manual", "set heater"}
  T35 = enum8{"Enabled", "Disabled", "Disabled and Grayed Out"}
  T36 = typedef "Set Point Aproach.ctl" = enum16{"Instant", "Ramp"}
  T37 = typedef "itc 503 box state.ctl" = cluster{"ITC503 Address":refnum<visa-resource-name>, "ITC temperature":dbl, "ITC set temperature":dbl, "heater":dbl, "gas flow":dbl, "P":dbl, "D":dbl, "I":dbl, "ITC state":string, "nonzero temperature":dbl, "Magn Field (T)":dbl}
  T38 = enum16{"check", "force UP", "stop UP/DOWN", "force DOWN", "init", "set gas to", "turn off", "turn on", "update parameters"}
  T39 = enum32{"Page Enabled", "Page Disabled", "Page Disabled & Grayed"}
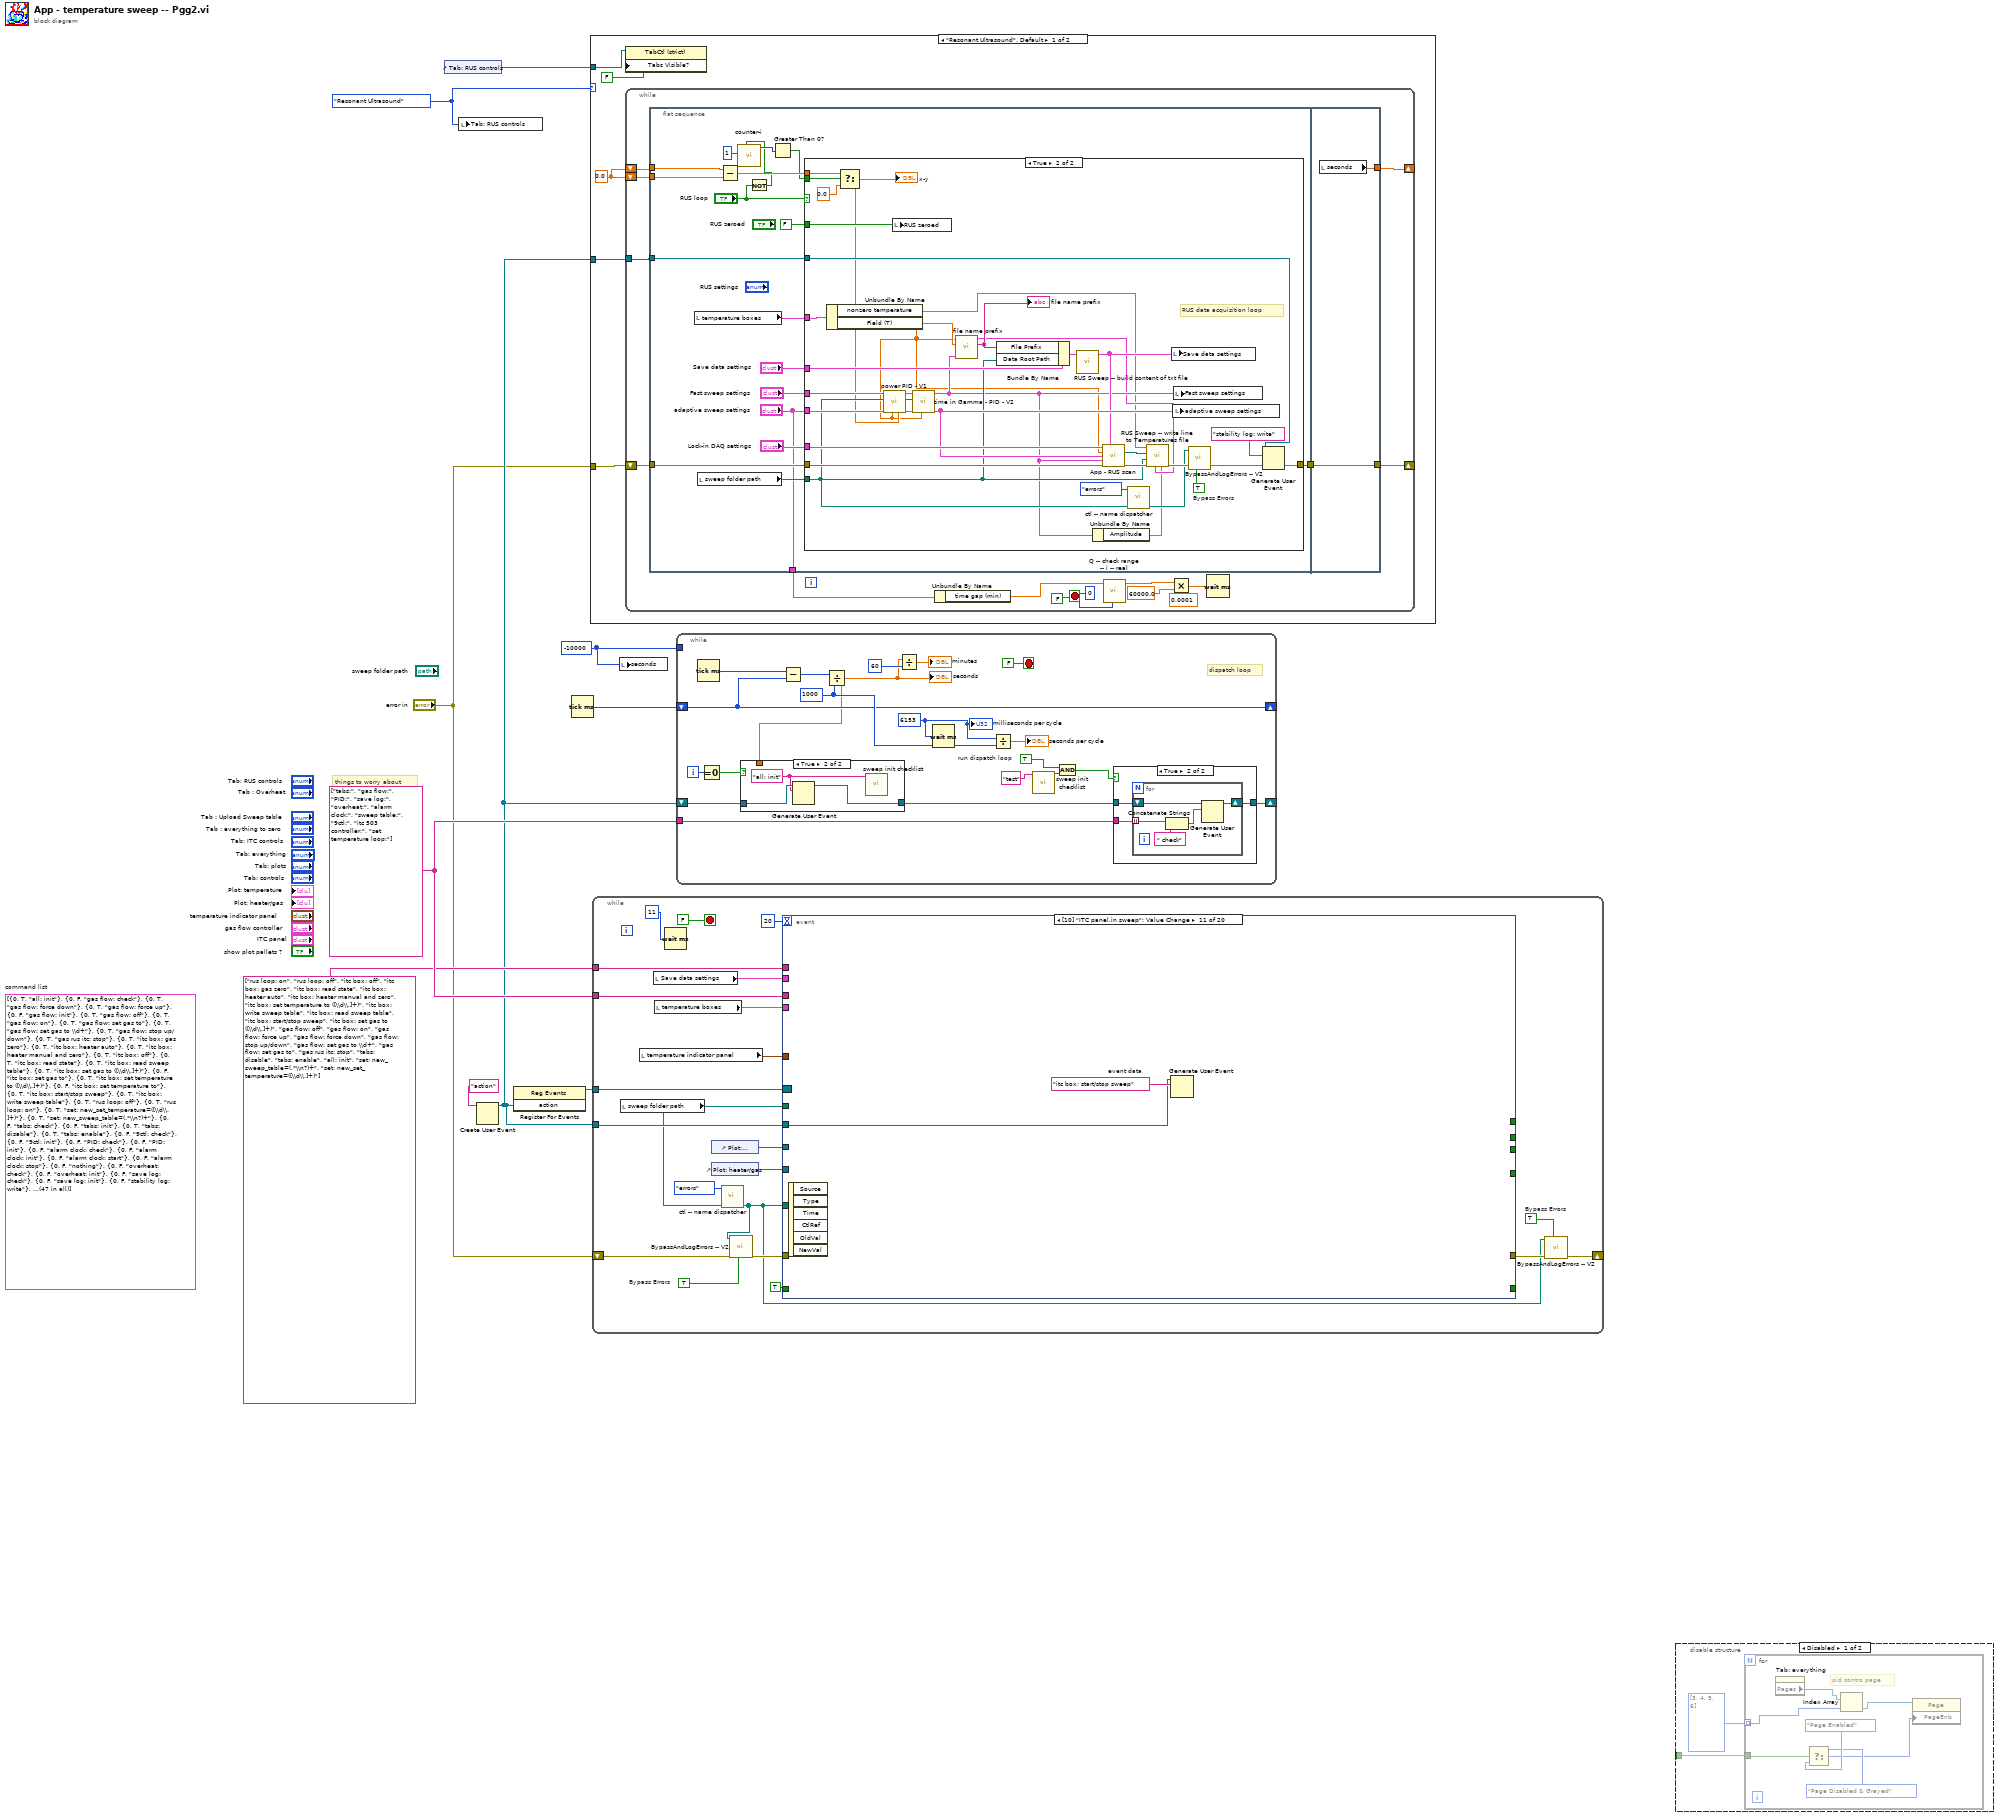
[diagram p0: block diagram]
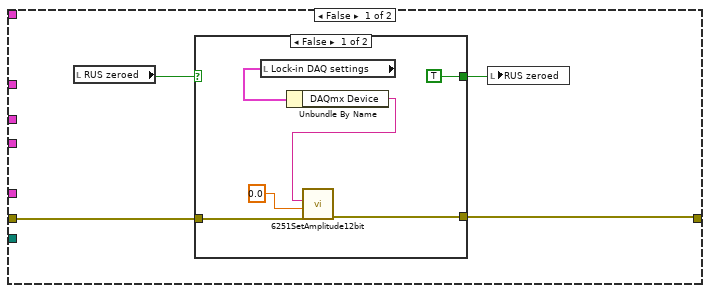
[diagram p2: hidden frame]
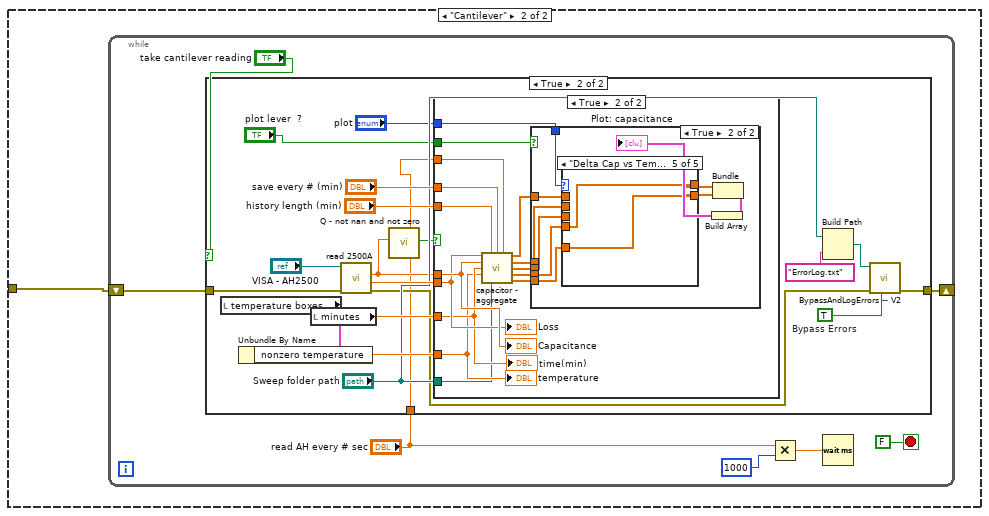
[diagram p4: hidden frame]
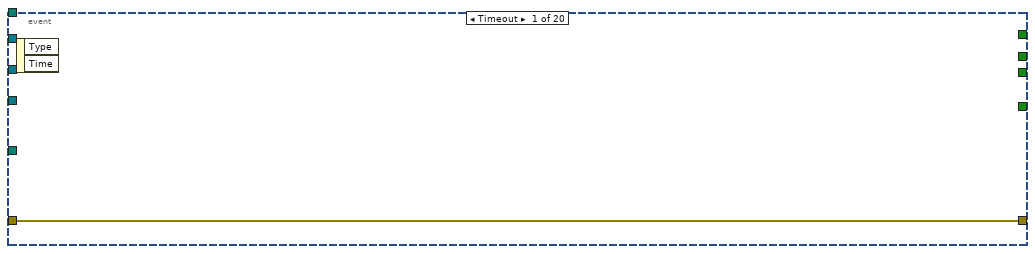
[diagram p13: hidden frame]
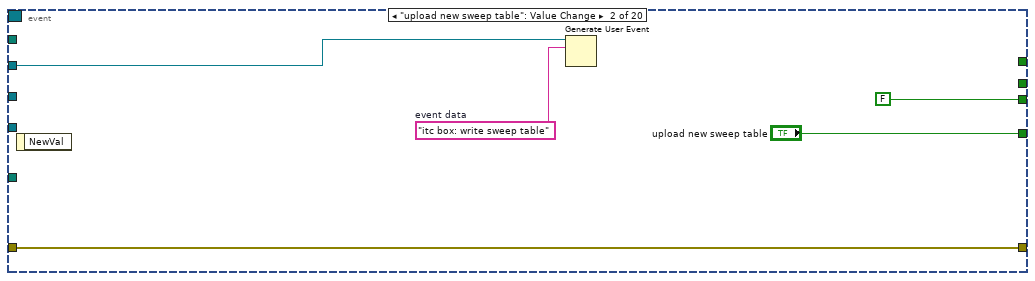
[diagram p14: hidden frame]
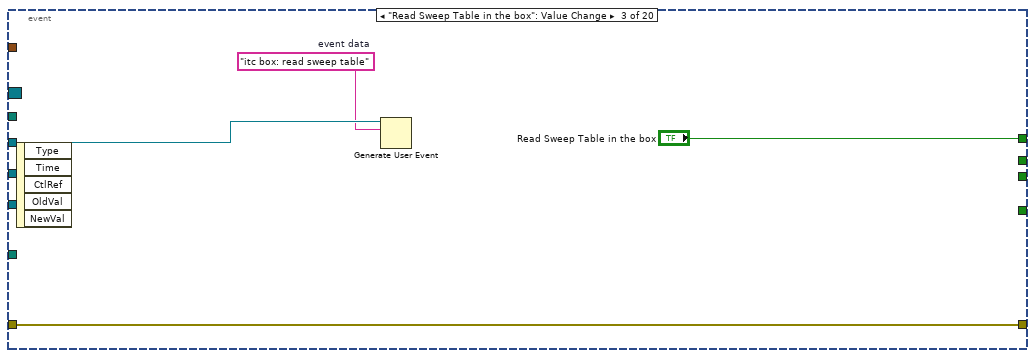
[diagram p15: hidden frame]
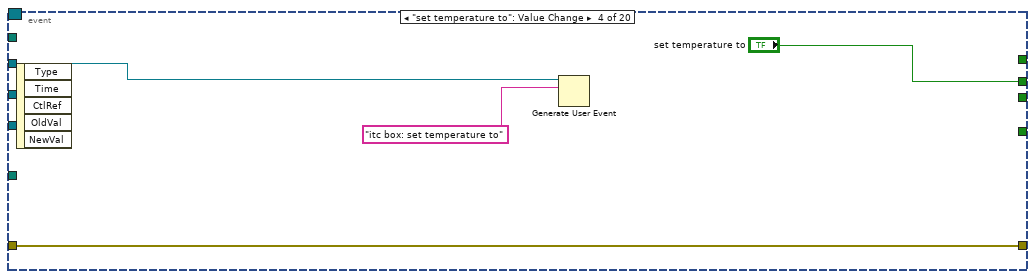
[diagram p16: hidden frame]
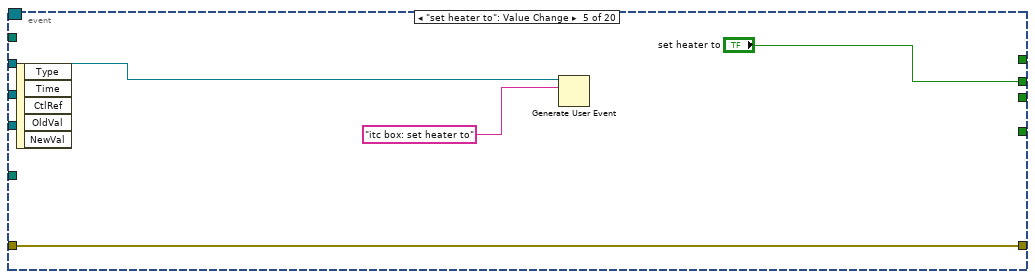
[diagram p17: hidden frame]
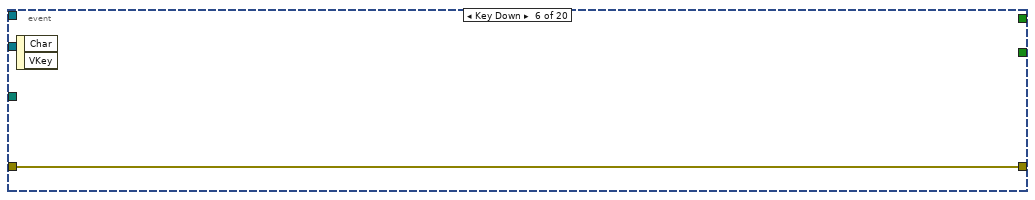
[diagram p18: hidden frame]
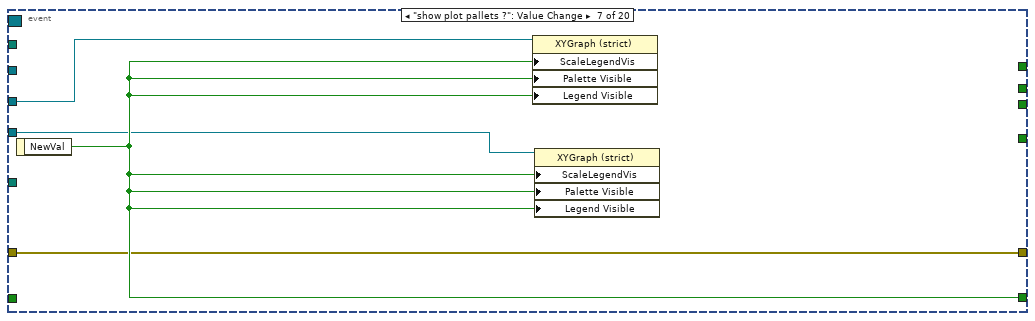
[diagram p19: hidden frame]
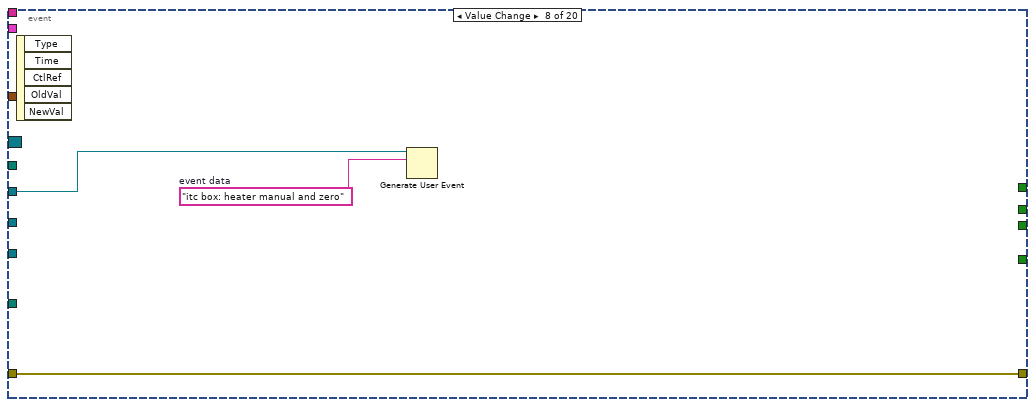
[diagram p20: hidden frame]
diagram:
  w1 = -10000 ("y")
  w2 = T2."Resonant Ultrasound" ("Tab: RUS controls")
  (unwired) T24[] [{"num"=0, "bool"=TRUE, "string"="all: init"}, {"num"=0, "bool"=FALSE, "string"="gas flow: check"}, {"num"=0, "bool"=TRUE, "string"="gas flow: force down"}, {"num"=0, "bool"=TRUE, "string"="gas flow: force up"}, {"num"=0, "bool"=FALSE, "string"="gas flow: init"}, {"num"=0, "bool"=TRUE, "string"="gas flow: off"}, {"num"=0, "bool"=TRUE, "string"="gas flow: on"}, {"num"=0, "bool"=TRUE, "string"="gas flow: set gas to"}, {"num"=0, "bool"=TRUE, "string"="gas flow: set gas to \\d+"}, {"num"=0, "bool"=TRUE, "string"="gas flow: stop up/down"}, {"num"=0, "bool"=TRUE, "string"="gas rus itc: stop"}, {"num"=0, "bool"=TRUE, "string"="itc box: gas zero"}, {"num"=0, "bool"=TRUE, "string"="itc box: heater auto"}, {"num"=0, "bool"=TRUE, "string"="itc box: heater manual and zero"}, {"num"=0, "bool"=TRUE, "string"="itc box: off"}, {"num"=0, "bool"=TRUE, "string"="itc box: read state"}, {"num"=0, "bool"=TRUE, "string"="itc box: read sweep table"}, {"num"=0, "bool"=TRUE, "string"="itc box: set gas to ([\\d\\.]+)"}, {"num"=0, "bool"=FALSE, "string"="itc box: set gas to"}, {"num"=0, "bool"=TRUE, "string"="itc box: set temperature to ([\\d\\.]+)"}, {"num"=0, "bool"=FALSE, "string"="itc box: set temperature to"}, {"num"=0, "bool"=TRUE, "string"="itc box: start/stop sweep"}, {"num"=0, "bool"=TRUE, "string"="itc box: write sweep table"}, {"num"=0, "bool"=TRUE, "string"="rus loop: off"}, {"num"=0, "bool"=TRUE, "string"="rus loop: on"}, {"num"=0, "bool"=TRUE, "string"="set: new_set_temperature=([\\d\\.]+)"}, {"num"=0, "bool"=TRUE, "string"="set: new_sweep_table=(.*\\n?)+"}, {"num"=0, "bool"=FALSE, "string"="tabs: check"}, {"num"=0, "bool"=FALSE, "string"="tabs: init"}, {"num"=0, "bool"=TRUE, "string"="tabs: disable"}, {"num"=0, "bool"=TRUE, "string"="tabs: enable"}, {"num"=0, "bool"=FALSE, "string"="9ctl: check"}, {"num"=0, "bool"=FALSE, "string"="9ctl: init"}, {"num"=0, "bool"=FALSE, "string"="PID: check"}, {"num"=0, "bool"=FALSE, "string"="PID: init"}, {"num"=0, "bool"=FALSE, "string"="alarm clock: check"}, {"num"=0, "bool"=FALSE, "string"="alarm clock: init"}, {"num"=0, "bool"=FALSE, "string"="alarm clock: start"}, {"num"=0, "bool"=FALSE, "string"="alarm clock: stop"}, {"num"=0, "bool"=FALSE, "string"="nothing"}, {"num"=0, "bool"=FALSE, "string"="overheat: check"}, {"num"=0, "bool"=FALSE, "string"="overheat: init"}, {"num"=0, "bool"=FALSE, "string"="save log: check"}, {"num"=0, "bool"=FALSE, "string"="save log: init"}, {"num"=0, "bool"=FALSE, "string"="stability log: write"}, {"num"=0, "bool"=FALSE, "string"="sweep table: init"}, {"num"=0, "bool"=FALSE, "string"="sweep table: check"}]  # command list
  w8 = string[] ["tabs:", "gas flow:", "PID:", "save log:", "overheat:", "alarm clock:", "sweep table:", "9ctl:", "itc 503 controller:", "set temperature loop:"]
  # "things to worry about"
  n1 = control-ref of="Tab: RUS controls"() -> (w6:refnum<vi>)
  n2 = local write "Tab: RUS controls"(w2) -> ()
  n3 = Create User Event(user event datatype="action" ("action")) -> (user event=w5:refnum<user-event>)  [unwired: 1 in, 1 out]
  n4 = register-events(w5) -> (reference out=w10:refnum<event-registration>)  [unwired: 2 in, 1 out]
  n5 = Tick Count (ms)() -> (millisecond timer value=w3:u32)
  n6 = case shown="\"Resonant Ultrasound\", Default" w2 {
    tunnel: "error in" -> [w15 w95]
    tunnel: w5 -> [w14 _]
    tunnel: w6 -> [w12 _]
    frame "Resonant Ultrasound", Default {
      w11 = 0.0
      n7 = property class="TabCtl (strict)"(reference=w12, "Tabs Visible?"=FALSE) -> ()  [unwired: 1 in, 2 out]
      n8 = while {
        shift-right: [w26] -> _
        shift-left: w15 -> [w29]
        tunnel: w14 -> [w24]
        shift-right: [w16] -> _
        shift-left: w11 -> [w19]
        shift-left: w11 -> [w18]
        stop <- FALSE stop-if-true
        (unwired) 0.0001
        n9 = flat-sequence {
          tunnel: w29 -> [w47]
          tunnel: w24 -> [w45]
          tunnel: ["adaptive sweep settings"] -> w21
          tunnel: w19 -> [w37]
          tunnel: w18 -> [w30]
          tunnel: [w46] -> w17
          tunnel: [w94] -> w26
          tunnel: w17 -> [w94]
          tunnel: [w93] -> w16
          frame #0 {
            n10 = local read "temperature boxes"() -> (w41:T21)
            n11 = local read "sweep folder path"() -> (w43:path)
            n12 = Subtract(x=w30, y=w37) -> (x-y=w36:dbl)
            n13 = Not(x="RUS loop") -> (.not. x?=w31:bool)
            n14 = call "counter-i.vi"("init ?"=w31, "cricket interval"=1) -> ("tic"=w34:i32)  [unwired: 8 in, 1 out]
            n15 = Greater Than 0?(x=w34) -> (x > 0?=w33:bool)
            n16 = case shown="True" "RUS loop" {
              tunnel: [w50 w83] -> w46
              tunnel: w47 -> [w51 w86]
              tunnel: w45 -> [_ w85]
              tunnel: FALSE ("frequency  format") -> [_ w81]
              tunnel: w43 -> [_ w69]
              tunnel: "Save data settings" -> [_ w77]
              tunnel: w41 -> [_ w76]
              tunnel: "Fast sweep settings" -> [_ w75]
              tunnel: "Lock-in DAQ settings" -> [_ w74]
              tunnel: "adaptive sweep settings" -> [_ w73]
              tunnel: w36 -> [_ w63]
              tunnel: w33 -> [_ w64]
              frame False {
                n17 = local read "RUS zeroed"() -> (w49:bool)
                n18 = case shown="False" w49 {
                  selector: w49 -> [_ w59]
                  tunnel: w51 -> [w56 w58]
                  tunnel: [w55 w58] -> w50
                  tunnel: [TRUE ("set amplitude to zero \nat end of every sweep") w59] -> w48
                  frame False {
                    n19 = local read "Lock-in DAQ settings"() -> (w54:T9)
                    n20 = Unbundle By Name(w54) -> ("DAQmx Device"=w53:tag)
                    n21 = call "6251SetAmplitude12bit.vi"("error in (no error)"=w56, "0 to 2.1 VRMS"=0.0, "DAQmx Device Name"=w53) -> ("error out"=w55:errorcluster)  [unwired: 8 out]
                  }
                  frame True {
                  }
                }
                n22 = local write "RUS zeroed"(w48) -> ()
              }
              frame True {
                w89 = TRUE  # Bypass Errors
                # "RUS data acquisition loop"
                n23 = Unbundle By Name(w76) -> ("nonzero temperature"=w60:dbl, "Field (T)"=w61:dbl)
                n24 = Select(t=w63, s=w64, f=0.0) -> (s? t:f=w65:dbl)
                "x-y" <- w65
                n25 = call "power PID - V1.vi"("delta time(sec)"=w65, "nonzero temperature"=w60, "adaptive sweep settings"=w73, "sweep folder path"=w69, "Fast sweep settings"=w75) -> ("adaptive sweep settings OUT"=w72:T3, "Fast sweep settings out"=w80:T6)  [unwired: 3 in, 2 out]
                n26 = local write "RUS zeroed"(w81) -> ()
                n27 = call "time in Gamma - PID - V2.vi"("nonzero temperature"=w60, "adaptive sweep settings"=w72, "sweep folder path"=w69, "Fast sweep settings"=w80) -> ("adaptive sweep settings OUT"=w71:T3, "Fast sweep settings out"=w68:T6)  [unwired: 4 in, 2 out]
                n28 = call "file name prefix.vi"("Fast sweep settings"=w68, "Magn Field (T)"=w61, "temperature"=w60) -> ("file name prefix"=w90:string, "filename cluster OUT"=w67:T26)  [unwired: 5 in, 2 out]
                "file name prefix" <- w90
                n29 = Bundle By Name(cluster=w77, "File Prefix"=w90, "Data Root Path"=w69) -> (w91:T7)
                n30 = call "RUS Sweep -- build content of txt file.vi"("Save data settings"=w91) -> ("Save data settings out"=w70:T7)  [unwired: 9 in, 1 out]
                n31 = Unbundle By Name(w68) -> ("Amplitude"=w66:dbl)
                n32 = call "App - RUS scan.vi"("Lock-in DAQ settings"=w74, "Save data settings"=w70, "temperature"=w60, "sweep settings"=w71, "Fast swep settings"=w68, "error in (no error)"=w86) -> ("Actual file path"=w92:path, "error out"=w87:errorcluster)  [unwired: 8 in]
                n33 = call "ctl -- name dispatcher.vi"("sweep folder path"=w69, "ctl name dispatch"=ctl_--_name_dispatcher_--_action."errors" ("ctl kind")) -> ("file path"=w78:path)  [unwired: 7 in, 2 out]
                n34 = call "RUS Sweep -- write line to Temperatures file.vi"("voltage"=w66, "filename cluster OUT"=w67, "error in"=w87, "sweep folder path"=w69, "file path"=w92, "LTC Temperature"=w60) -> ("error out"=w88:errorcluster)  [unwired: 5 in]
                n35 = local write "Save data settings"(w70) -> ()
                n36 = local write "adaptive sweep settings"(w71) -> ()
                n37 = local write "Fast sweep settings"(w68) -> ()
                n38 = call "BypassAndLogErrors -- V2.vi"("Bypass Errors"=w89, "error in (no error)"=w88, "Log File Path"=w78) -> ("error out"=w82:errorcluster)  [unwired: 8 in]
                n39 = Generate User Event(user event=w85, event data cluster="stability log: write" ("name or relative path"), error in=w82) -> (error out=w83:errorcluster)  [unwired: 1 in, 1 out]
              }
            }
          }
          frame #1 {
            n40 = local read "seconds"() -> (w93:dbl)
          }
        }
        n41 = Unbundle By Name(w21) -> ("time gap (min)"=w20:dbl)
        n42 = call "Q -- check range -- i -- real.vi"("lower"=0, "number"=w20) -> ("number in range"=w22:dbl)  [unwired: 7 in, 2 out]
        n43 = Multiply(x=w22, y=60000.0) -> (x*y=w28:dbl)
        n44 = Wait (ms)(milliseconds to wait=w28) -> ()  [unwired: 1 out]
      }
    }
    frame "Cantilever" {
      n45 = while {
        shift-right: [w99] -> _
        shift-left: w95 -> [w100]
        stop <- FALSE ("Boolean") stop-if-true
        n46 = case shown="True" "take cantilever reading" {
          tunnel: w100 -> [w103 w111]
          tunnel: [w103 w109] -> w99
          tunnel: "read AH every # sec" -> [_ w104]
          frame False {
          }
          frame True {
            w115 = TRUE  # Bypass Errors
            n47 = local read "temperature boxes"() -> (w117:T21)
            n48 = Unbundle By Name(w117) -> ("nonzero temperature"=w116:dbl)
            n49 = local read "minutes"() -> (w118:dbl)
            n50 = call "read 2500A.vi"("error in (no error)"=w111, "VISA Resource Name"="VISA - AH2500") -> ("error out"=w110:errorcluster, "Loss"=w119:dbl, "Capacitance"=w108:dbl)  [unwired: 6 in, 1 out]
            n51 = call "Q - not nan and not zero.vi"("Numeric"=w108) -> ("Boolean"=w107:bool)  [unwired: 10 in]
            n52 = case shown="True" w107 {
              tunnel: "history length (min)" -> [_ w137]
              tunnel: "save every # (min)" -> [_ w136]
              tunnel: w104 -> [_ w135]
              tunnel: w108 -> [_ w134]
              tunnel: w119 -> [_ w133]
              tunnel: w118 -> [_ w132]
              tunnel: w116 -> [_ w131]
              tunnel: "Sweep folder path" -> [_ w126]
              tunnel: "plot" -> [_ w124]
              tunnel: "plot lever  ?" -> [_ w123]
              frame False {
              }
              frame True {
                n53 = call "capacitor - aggregate.vi"("loss"=w133, "history length (min)"=w137, "save every # (min)"=w136, "aggregate every # sec"=w135, "capacitance"=w134, "time(min)"=w132, "temperature"=w131, "Sweep folder path"=w126) -> ("loss array"=w127:dbl[], "capacitance array"=w130:dbl[], "time(min) array"=w129:dbl[], "temperature array"=w128:dbl[], "delta capacitance array"=w125:dbl[])  [unwired: 3 in]
                n54 = case shown="True" w123 {
                  tunnel: w130 -> [_ w144]
                  tunnel: w129 -> [_ w142]
                  tunnel: w128 -> [_ w141]
                  tunnel: w127 -> [_ w140]
                  tunnel: w125 -> [_ w139]
                  tunnel: w124 -> [_ w138]
                  frame False {
                  }
                  frame True {
                    n55 = case shown="\"Delta Cap vs Temp\"" w138 {
                      tunnel: [w149 w151 w153 w155 w156] -> w145
                      tunnel: w144 -> [w149 w151 _ _ _]
                      tunnel: [w148 w150 w152 w154 w157] -> w143
                      tunnel: w142 -> [w148 _ w152 _ _]
                      tunnel: w141 -> [_ w150 _ w154 w157]
                      tunnel: w140 -> [_ _ w153 w155 _]
                      tunnel: w139 -> [_ _ _ _ w156]
                      frame "Capac vs Time", Default {
                      }
                      frame "Capac vs Temp" {
                      }
                      frame "Loss  vs Time" {
                      }
                      frame "Loss vs Temp" {
                      }
                      frame "Delta Cap vs Temp" {
                      }
                    }
                    n56 = Bundle("temperature array"=w143, "delta capacitance array"=w145) -> (w147:T27)  [unwired: 1 in]
                    n57 = Build Array(w147) -> (→"Plot: capacitance":T28)
                  }
                }
                "Loss" <- w133
                "Capacitance" <- w134
                "time(min)" <- w132
                "temperature" <- w131
              }
            }
            n58 = Build Path(base path="Sweep folder path", name or relative path="ErrorLog.txt") -> (appended path=w112:path)
            n59 = call "BypassAndLogErrors -- V2.vi"("Bypass Errors"=w115, "error in (no error)"=w110, "Log File Path"=w112) -> ("error out"=w109:errorcluster)  [unwired: 8 in]
          }
        }
        n60 = Multiply(x="read AH every # sec", y=1000) -> (x*y=w97:dbl)
        n61 = Wait (ms)(milliseconds to wait=w97) -> ()  [unwired: 1 out]
      }
    }
  }
  n62 = while {
    shift-right: [w161] -> _
    shift-left: "error in" -> [w167]
    tunnel: w10 -> [w177]
    tunnel: w5 -> [w176]
    tunnel: w8 -> [w170]
    tunnel: string[] ["rus loop: on", "rus loop: off", "itc box: off", "itc box: gas zero", "itc box: read state", "itc box: heater auto", "itc box: heater manual and zero", "itc box: set temperature to ([\\d\\.]+)", "itc box: write sweep table", "itc box: read sweep table", "itc box: start/stop sweep", "itc box: set gas to ([\\d\\.]+)", "gas flow: off", "gas flow: on", "gas flow: force up", "gas flow: force down", "gas flow: stop up/down", "gas flow: set gas to \\d+", "gas flow: set gas to", "gas rus itc: stop", "tabs: disable", "tabs: enable", "all: init", "set: new_sweep_table=(.*\\n?)+", "set: new_set_temperature=([\\d\\.]+)"] -> [w165]
    stop <- FALSE stop-if-true
    w163 = TRUE  # Bypass Errors
    w168 = TRUE  # Bypass Errors
    n63 = local read "sweep folder path"() -> (w158:path)
    n64 = local read "temperature indicator panel"() -> (w171:T19)
    n65 = local read "Save data settings"() -> (w164:T7)
    n66 = local read "temperature boxes"() -> (w172:T21)
    n67 = Wait (ms)(milliseconds to wait=u32 11 ("milliseconds per cycle")) -> ()  [unwired: 1 out]
    n68 = control-ref of="Plot: temperature"() -> (w174:refnum<vi>)
    n69 = control-ref of="Plot: heater/gas"() -> (w175:refnum<vi>)
    n70 = call "ctl -- name dispatcher.vi"("sweep folder path"=w158, "ctl name dispatch"=ctl_--_name_dispatcher_--_action."errors" ("ctl kind")) -> ("file path"=w159:path)  [unwired: 7 in, 2 out]
    n71 = call "BypassAndLogErrors -- V2.vi"("Bypass Errors"=w168, "error in (no error)"=w167, "Log File Path"=w159) -> ("error out"=w166:errorcluster)  [unwired: 8 in]
    n72 = event shown="[10] \"ITC panel.in sweep\": Value Change" {
      selector: w177 -> [_ _ _ _ _ _ _ _ _ _ _ _ _ _ _ _ _ _ _ _]
      dyn-events: _ -> [_ _ _ _ _ _ _ _ _ _ _ _ _ _ _ _ _ _ _ _]
      timeout: 20 -> [_ _ _ _ _ _ _ _ _ _ _ _ _ _ _ _ _ _ _ _]
      tunnel: [_ "upload new sweep table" _ _ _ _ _ _ _ _ _ _ _ _ _ _ _ _ _ _] -> _
      tunnel: w166 -> [w180 w181 w186 w192 w197 w198 w199 w203 w208 w216 _ w1102 w1111 w1112 w1115 w1118 w1121 w1130 w1131 w1134]
      tunnel: [w180 w181 w186 w192 w197 w198 w199 w203 w208 w212 _ w1102 w1111 w1112 w1115 w1118 w1121 w1130 w1131 w1134] -> w162
      tunnel: [_ FALSE _ _ _ _ _ _ _ _ _ _ _ _ _ _ _ _ _ _] -> _
      tunnel: [_ _ "Read Sweep Table in the box" _ _ _ _ _ _ _ _ _ _ _ _ _ _ _ _ _] -> _
      tunnel: [_ _ _ "set temperature to" "set heater to" _ _ _ _ _ _ _ _ _ _ _ _ _ _ _] -> _
      tunnel: [_ _ _ _ _ _ w202 _ _ _ _ _ _ _ _ _ _ _ _ _] -> _
      tunnel: TRUE -> [_ _ _ _ _ _ _ _ _ _ _ _ _ _ _ _ _ _ _ _]
      tunnel: w176 -> [_ w182 w188 w191 w196 _ _ w205 w207 w222 w1096 _ w1110 w1114 w1116 w1119 w1126 _ w1133 w1136]
      tunnel: w175 -> [_ _ _ _ _ _ w201 _ _ _ _ _ _ _ _ _ _ _ _ _]
      tunnel: w174 -> [_ _ _ _ _ _ w200 _ _ _ _ _ _ _ _ _ _ _ _ _]
      tunnel: w164 -> [_ _ _ _ _ _ _ _ _ _ _ w1107 _ _ _ _ _ _ _ _]
      tunnel: w172 -> [_ _ _ _ _ _ _ _ _ w220 _ w1104 _ _ _ _ _ _ _ _]
      tunnel: w171 -> [_ _ _ _ _ _ _ _ _ w219 _ _ _ _ _ _ _ _ _ _]
      tunnel: w170 -> [_ _ _ _ _ _ _ _ _ w218 _ _ _ _ _ _ _ _ _ _]
      tunnel: w165 -> [_ _ _ _ _ _ _ _ _ w215 _ _ _ _ _ _ _ _ _ _]
      tunnel: w159 -> [_ _ _ _ _ _ _ _ _ w209 _ _ _ _ _ _ _ _ _ _]
      tunnel: w158 -> [_ _ _ _ _ _ _ _ _ w211 _ _ _ _ _ _ _ _ _ _]
      event Timeout {
        n73 = event-data() -> ()  [unwired: 1 in, 2 out]
      }
      event "upload new sweep table": Value Change {
        w183 = "itc box: write sweep table"  # event data
        n74 = event-data() -> ()  [unwired: 1 in, 1 out]
        n75 = Generate User Event(user event=w182, event data cluster=w183) -> ()  [unwired: 2 in, 2 out]
      }
      event "Read Sweep Table in the box": Value Change {
        w187 = "itc box: read sweep table"  # event data
        n76 = event-data() -> ()  [unwired: 1 in, 5 out]
        n77 = Generate User Event(user event=w188, event data cluster=w187) -> ()  [unwired: 2 in, 2 out]
      }
      event "set temperature to": Value Change {
        n78 = event-data() -> ()  [unwired: 1 in, 5 out]
        n79 = Generate User Event(user event=w191, event data cluster="itc box: set temperature to" ("action")) -> ()  [unwired: 2 in, 2 out]
      }
      event "set heater to": Value Change {
        n80 = event-data() -> ()  [unwired: 1 in, 5 out]
        n81 = Generate User Event(user event=w196, event data cluster="itc box: set heater to" ("action")) -> ()  [unwired: 2 in, 2 out]
      }
      event Key Down {
        n82 = event-data() -> ()  [unwired: 1 in, 2 out]
      }
      event "show plot pallets ?": Value Change {
        n83 = event-data() -> ("NewVal"=w202:bool)  [unwired: 1 in]
        n84 = property on="Property Node" class="XYGraph (strict)"(reference=w200, "ScaleLegendVis"=w202, "Palette Visible"=w202, "Legend Visible"=w202) -> ()  [unwired: 1 in, 2 out]
        n85 = property on="Property Node" class="XYGraph (strict)"(reference=w201, "ScaleLegendVis"=w202, "Palette Visible"=w202, "Legend Visible"=w202) -> ()  [unwired: 1 in, 2 out]
      }
      event Value Change {
        w204 = "itc box: heater manual and zero"  # event data
        n86 = event-data() -> ()  [unwired: 1 in, 5 out]
        n87 = Generate User Event(user event=w205, event data cluster=w204) -> ()  [unwired: 2 in, 2 out]
      }
      event Value Change {
        w206 = "itc box: heater auto"  # event data
        n88 = event-data() -> ()  [unwired: 1 in, 5 out]
        n89 = Generate User Event(user event=w207, event data cluster=w206) -> ()  [unwired: 2 in, 2 out]
      }
      event User Event {
        n90 = event-data() -> ("action"=w223:string)  [unwired: 1 in]
        n91 = local read "seconds per cycle"() -> (w213:dbl)
        n92 = local read "seconds"() -> (w214:dbl)
        n93 = case shown="\"itc box: start/stop sweep\"" w223 {
          selector: w223 -> [_ w243 _ w273 _ w293 w299 w305 w310 _ _ _ w347 _ _ _ _ _ _ _ _ _ _ _ _ _ _ _ _ w456 _ w975 _ _ _ w992 _ w1008 _ w1036 _ _ _ _ w1055 w1058 w1066]
          tunnel: w214 -> [_ _ w255 _ w277 w289 w294 w300 _ w328 _ _ w342 _ _ _ _ _ _ _ _ _ _ _ _ _ _ _ _ _ _ _ _ _ w985 w990 _ _ w1024 _ _ _ _ _ _ _ _]
          tunnel: w222 -> [w227 _ _ _ w283 _ _ _ w307 _ _ _ _ _ _ _ _ w358 _ _ _ _ _ _ _ _ _ _ w436 w451 w958 _ _ _ _ _ _ _ _ _ _ _ _ _ _ _ _]
          tunnel: FALSE -> [_ _ _ _ _ _ _ _ _ _ _ _ _ _ _ _ _ _ _ _ _ _ _ _ _ _ _ _ _ _ _ w976 w978 _ _ _ _ _ _ _ _ _ _ _ _ _ _]
          tunnel: w220 -> [_ _ w256 w271 _ _ _ _ _ w327 _ _ w344 _ _ _ _ _ _ _ _ _ w393 _ _ _ _ _ _ _ w960 _ _ _ w984 _ w996 _ w1025 _ _ _ _ _ _ _ w1059]
          tunnel: w219 -> [_ _ _ _ _ _ _ _ _ w325 _ _ w343 _ _ _ _ _ _ _ _ _ _ _ _ _ _ _ _ _ _ _ _ _ _ _ _ _ _ _ _ _ _ _ _ _ _]
          tunnel: w218 -> [_ _ _ _ _ _ _ _ w309 _ _ _ _ _ _ _ _ _ _ _ _ _ _ _ _ _ _ _ _ _ _ _ _ _ _ _ _ _ _ _ _ _ _ _ _ _ _]
          tunnel: TRUE -> [_ _ _ _ _ _ _ _ _ _ _ _ _ _ _ _ _ _ _ _ _ _ _ _ _ _ _ _ _ _ _ _ _ w980 _ _ _ _ _ _ _ _ _ _ _ _ _]
          tunnel: w216 -> [w226 w242 w254 w272 w281 w292 w298 w304 w306 w323 w336 w338 w341 w349 w351 w353 w355 w356 w364 w366 w369 w372 w383 w401 w408 w411 w415 w419 w437 w452 w956 w974 w977 w979 w983 w991 w995 w1010 w1022 w1035 w1039 w1040 w1041 w1046 w1051 w1057 w1065]
          tunnel: [w226 w242 w253 w272 w281 w292 w298 w304 w306 w323 w336 w338 w341 w349 w351 w353 w355 w356 w363 w365 w368 w371 w383 w397 w407 w410 w414 w418 w434 w452 w956 w974 w977 w979 w983 w991 w995 w1009 w1021 w1035 w1039 w1040 w1041 w1046 w1051 w1057 w1064] -> w212
          tunnel: w215 -> [w225 _ _ _ _ _ _ _ _ _ _ _ _ _ _ _ _ _ _ _ _ _ _ _ _ _ _ _ _ _ _ _ _ _ _ _ _ _ _ _ _ _ _ _ _ _ _]
          tunnel: w213 -> [_ _ _ _ _ _ _ _ _ _ _ _ _ _ _ _ _ _ _ _ _ _ _ _ _ _ _ _ _ _ _ _ _ _ _ _ _ _ w1023 _ _ _ _ _ _ _ w1062]
          tunnel: w211 -> [_ w238 w248 _ _ _ _ _ _ _ _ _ _ _ _ _ _ _ _ _ _ _ _ _ _ _ _ _ _ _ _ _ _ _ w981 _ w994 w1006 _ _ _ _ _ _ _ _ w1063]
          tunnel: "interaction with itc" -> [_ _ _ _ _ _ _ _ _ _ _ _ _ _ _ _ _ _ _ _ _ _ _ _ _ _ _ _ _ _ _ _ _ _ _ _ _ w1004 w1020 _ _ _ _ _ _ _ _]
          tunnel: w209 -> [_ _ _ _ _ _ _ _ _ _ _ _ _ _ _ _ _ _ _ _ _ _ _ _ _ _ _ _ _ _ _ _ _ _ _ _ _ _ w1019 _ _ _ _ _ _ _ _]
          frame "9ctl: check" {
            # "list of commands understood by protocol"
            n94 = call "p9ctl.vi"("p9 action"=p9action_control."check") -> ("ctl"=w229:string, "news?"=w228:bool)  [unwired: 8 in, 1 out]
            n95 = case shown="True" w228 {
              tunnel: w229 -> [_ w231]
              tunnel: w227 -> [_ w232]
              tunnel: w225 -> [_ w235]
              frame False {
              }
              frame True {
                n96 = call "test for a regexp list.vi"("quote specials"=FALSE, "string"=w231, "regexps"=w235) -> ("whole match"=w230:string, "match found"=w233:bool)  [unwired: 5 in, 2 out]
                n97 = case shown="True" w233 {
                  tunnel: w232 -> [_ w237]
                  tunnel: w230 -> [_ w236]
                  frame False {
                  }
                  frame True {
                    n98 = Generate User Event(user event=w237, event data cluster=w236) -> ()  [unwired: 2 in, 2 out]
                  }
                }
              }
            }
          }
          frame "9ctl: init" {
            (unwired) path "C:/THIS_FOLDER_DOES_NOT_EXIST"  # ctl path
            w239 = path "C:/Users/riggslab/Desktop/arkady/Dropbox/ultrasound_experiment/9ctl"  # ctl path
            n99 = call "sweep init checklist.vi"("action"=w243) -> ()  [unwired: 10 in, 1 out]
            n100 = call "p9ctl.vi"("p9 action"=p9action_control."init", "ctl path"=w239, "sweep folder path"=w238) -> ("9ctl OK"=→"9ctl OK":bool)  [unwired: 6 in, 2 out]
          }
          frame "PID: check" {
            n101 = Unbundle By Name(w256) -> ("ITC temperature"=w247:dbl)
            n102 = control-ref of="PID timer"() -> (w251:refnum<vi>)
            n103 = call "slider timer .vi"("interval (sec)"=100.0, "action"=countdown_control."check", "timer ref"=w251) -> ("tic"=w250:bool)  [unwired: 6 in, 2 out]
            n104 = call "Q -- check range -- i -- real.vi"("lower"=0.01, "number"=w247) -> ("in range?"=w245:bool)  [unwired: 7 in, 2 out]
            n105 = And(x=w245, y=w250) -> (x .and. y?=w249:bool)
            n106 = case shown="True" w249 {
              tunnel: w255 -> [_ _]
              tunnel: w247 -> [_ w264]
              tunnel: w254 -> [w257 w263]
              tunnel: [w257 w262] -> w253
              tunnel: w248 -> [_ w260]
              frame False {
              }
              frame True {
                w261 = enum16{"CHECK", "INIT"}."CHECK"  # action
                n107 = call "Control PID -- Pgg1.vi"("action"=w261, "ITC temperature"=w264, "error in"=w263, "sweep folder path"=w260) -> ("error out"=w262:errorcluster, "PID"=→"PID":dbl[], "OK?"=→"PID OK":bool)  [unwired: 5 in]
                "PID temperature" <- w264
              }
            }
          }
          frame "PID: init" {
            w265 = countdown_control."start" ("action")
            w270 = enum16{"CHECK", "INIT"}."INIT"  # action
            n108 = Unbundle By Name(w271) -> ("ITC temperature"=w269:dbl)
            n109 = call "sweep init checklist.vi"("action"=w273) -> ()  [unwired: 10 in, 1 out]
            n110 = control-ref of="PID timer"() -> (w268:refnum<vi>)
            n111 = call "slider timer .vi"("interval (sec)"=100.0, "action"=w265, "timer ref"=w268) -> ("timer out"=w266:refnum<vi>)  [unwired: 6 in, 2 out]
            n112 = call "slider timer .vi"("action"=w265, "timer ref"=w266) -> ()  [unwired: 7 in, 3 out]
            n113 = call "Control PID -- Pgg1.vi"("action"=w270, "ITC temperature"=w269) -> ()  [unwired: 7 in, 3 out]
          }
          frame "alarm clock: check" {
            w280 = enum16{"init", "check", "start", "stop"}."check"  # action
            n114 = call "alarm clock - fancy.vi"("action"=w280, "alarm"="alarm", "seconds"=w277) -> ("alarm out"=w278:T20, "alarm!"=w276:bool)  [unwired: 7 in]
            n115 = And(x=w276, y=FALSE) -> (x .and. y?=w274:bool)
            n116 = case shown="True" w274 {
              tunnel: w283 -> [_ w285]
              tunnel: string[] ["gas flow: off", "rus loop: off", "itc box: off"] -> [_ w284]
              frame False {
              }
              frame True {
                n117 = for {
                  tunnel: w285 -> [w287]
                  tunnel: w284 -> [w286] mode=indexing
                  n118 = Generate User Event(user event=w287, event data cluster=w286) -> ()  [unwired: 2 in, 2 out]
                }
              }
            }
            n119 = local write "alarm"(w278) -> ()
          }
          frame "alarm clock: init" {
            w288 = enum16{"init", "check", "start", "stop"}."init"  # action
            n120 = local read "alarm"() -> (w291:T20)
            n121 = call "sweep init checklist.vi"("action"=w293) -> ()  [unwired: 10 in, 1 out]
            n122 = call "alarm clock - fancy.vi"("action"=w288, "alarm"=w291, "seconds"=w289) -> ("alarm out"=w290:T20)  [unwired: 7 in, 1 out]
            n123 = local write "alarm"(w290) -> ()
          }
          frame "alarm clock: start" {
            w297 = enum16{"init", "check", "start", "stop"}."start"  # action
            n124 = local read "alarm"() -> (w296:T20)
            n125 = call "sweep init checklist.vi"("action"=w299) -> ()  [unwired: 10 in, 1 out]
            n126 = call "alarm clock - fancy.vi"("action"=w297, "alarm"=w296, "seconds"=w294) -> ("alarm out"=w295:T20)  [unwired: 7 in, 1 out]
            n127 = local write "alarm"(w295) -> ()
          }
          frame "alarm clock: stop" {
            w303 = enum16{"init", "check", "start", "stop"}."stop"  # action
            n128 = local read "alarm"() -> (w302:T20)
            n129 = call "sweep init checklist.vi"("action"=w305) -> ()  [unwired: 10 in, 1 out]
            n130 = call "alarm clock - fancy.vi"("action"=w303, "alarm"=w302, "seconds"=w300) -> ("alarm out"=w301:T20)  [unwired: 7 in, 1 out]
            n131 = local write "alarm"(w301) -> ()
          }
          frame "all: init" {
            n132 = for {
              tunnel: w309 -> [w313] mode=indexing
              tunnel: [w311] -> w308 mode=indexing
              n133 = Concatenate Strings(w313, " init" ("event data")) -> (w311:string)
            }
            n134 = call "sweep init checklist.vi"("list"=w308, "init str"=w310, "action"=w310) -> ()  [unwired: 8 in, 1 out]
            n135 = for {
              tunnel: w307 -> [w315]
              tunnel: w308 -> [w314] mode=indexing
              n136 = Generate User Event(user event=w315, event data cluster=w314) -> ()  [unwired: 2 in, 2 out]
            }
          }
          frame "gas flow: check" {
            n137 = Unbundle By Name(w325) -> ("heater i-average, V"=w324:dbl)
            n138 = Unbundle By Name(w327) -> ("gas flow"=w326:dbl)
            n139 = call "gas flow controller -- Pgg3.vi"("gas flow, %"=w326, "action"=gas_flow_controller_action."check", "heater"=w324, "seconds"=w328) -> ("gas flow controller out"=w316:T17)  [unwired: 7 in]
            n140 = Unbundle By Name(w316) -> ("ramp Up progress"=→"ramp Up progress":T18, "ramp Down progress"=→"ramp Down progress":T18, "state"=w319:enum16{"normal", "ramp up", "ramp down"})
            n141 = case shown="\"ramp down\"" w319 {
              tunnel: [FALSE TRUE FALSE] -> w318
              tunnel: [TRUE FALSE FALSE] -> w317
              frame "ramp up" {
              }
              frame "ramp down" {
              }
              frame "normal", Default {
              }
            }
            n142 = property on="ramp Up progress" class="Clust (strict)"("Visible"=w317) -> ()  [unwired: 2 in, 2 out]
            n143 = property on="ramp Down progress" class="Clust (strict)"("Visible"=w318) -> ()  [unwired: 2 in, 2 out]
          }
          frame "gas flow: force down" {
            n144 = call "gas flow controller -- Pgg3.vi"("action"=gas_flow_controller_action."force DOWN") -> ()  [unwired: 10 in, 1 out]
          }
          frame "gas flow: force up" {
            n145 = call "gas flow controller -- Pgg3.vi"("action"=gas_flow_controller_action."force UP") -> ()  [unwired: 10 in, 1 out]
          }
          frame "gas flow: init" {
            n146 = control-ref of="gas flow controller"() -> (w339:refnum<vi>)
            n147 = Unbundle By Name(w344) -> ("heater"=w345:dbl, "gas flow"=w346:dbl)
            n148 = Unbundle By Name(w343) -> ()  [unwired: 1 out]
            n149 = call "sweep init checklist.vi"("action"=w347) -> ()  [unwired: 10 in, 1 out]
            n150 = call "gas flow controller -- Pgg3.vi"("gas flow, %"=w346, "action"=gas_flow_controller_action."init", "heater"=w345, "gas flow controller ref in"=w339, "seconds"=w342) -> ()  [unwired: 6 in, 1 out]
          }
          frame "gas flow: off" {
            n151 = call "gas flow controller -- Pgg3.vi"("action"=gas_flow_controller_action."turn off") -> ()  [unwired: 10 in, 1 out]
          }
          frame "gas flow: on" {
            n152 = call "gas flow controller -- Pgg3.vi"("action"=gas_flow_controller_action."turn on") -> ()  [unwired: 10 in, 1 out]
          }
          frame "gas flow: set gas to" {
            n153 = call "gas flow controller -- Pgg3.vi"("action"=gas_flow_controller_action."set gas to") -> ()  [unwired: 10 in, 1 out]
          }
          frame "gas flow: stop up/down" {
            n154 = call "gas flow controller -- Pgg3.vi"("action"=gas_flow_controller_action."stop UP/DOWN") -> ()  [unwired: 10 in, 1 out]
          }
          frame "gas rus itc: stop" {
            n155 = for {
              tunnel: w358 -> [w360]
              tunnel: string[] ["gas flow: off", "rus loop: off", "itc box: off"] -> [w359] mode=indexing
              n156 = Generate User Event(user event=w360, event data cluster=w359) -> ()  [unwired: 2 in, 2 out]
            }
          }
          frame "itc box: gas zero" {
            w361 = itc_503_box_-_control."set gas to"  # itc box action
            w362 = 1.0  # Gas %
            n157 = call "itc Hg box controller -- wrapper -- A1.vi"("itc box action"=w361, "error in"=w364, "input"=w362) -> ("error out"=w363:errorcluster)  [unwired: 6 in, 2 out]
          }
          frame "itc box: heater auto" {
            w367 = itc_503_box_-_control."heater auto"  # itc box action
            n158 = call "itc Hg box controller -- wrapper -- A1.vi"("itc box action"=w367, "error in"=w366) -> ("error out"=w365:errorcluster)  [unwired: 7 in, 2 out]
          }
          frame "itc box: heater manual and zero" {
            w370 = itc_503_box_-_control."heater manual and zero"  # itc box action
            n159 = call "itc Hg box controller -- wrapper -- A1.vi"("itc box action"=w370, "error in"=w369) -> ("error out"=w368:errorcluster)  [unwired: 7 in, 2 out]
          }
          frame "itc box: off" {
            w373 = itc_503_box_-_control."shut off"  # itc box action
            n160 = call "itc Hg box controller -- wrapper -- A1.vi"("itc box action"=w373, "error in"=w372) -> ("error out"=w371:errorcluster)  [unwired: 7 in, 2 out]
          }
          frame "itc box: read state" {
            (unwired) "\nsweeptable=\n"
            n161 = local read "date string Array"() -> (w376:string[])
            n162 = local read "Sweep Table"() -> (w377:dbl[][])
            n163 = Unbundle By Name(w393) -> ("ITC temperature"=w392:dbl, "ITC set temperature"=w375:dbl, "LTC temperature"=w391:dbl, "heater"=w390:dbl, "gas flow"=w389:dbl, "P"=w388:dbl, "D"=w387:dbl, "I"=w386:dbl, "ITC state"=w385:string, "nonzero temperature"=w379:dbl)
            n164 = call "string -- format sweep table string.vi"("ITC set temperature"=w375, "date string Array"=w376, "Sweep Table"=w377) -> ("string out"=w374:string)  [unwired: 8 in]
            n165 = Format Into String(format string="itc=%4f  itc_set=%4f  ltc=%4f  heater=%3f  gas=%3f  P=%3f  D=%3f  I=%3f  itc_state=%s  nzt=%3f" ("action"), w392, w375, w391, w390, w389, w388, w387, w386, w385, w379) -> (resulting string=w382:string)  [unwired: 2 in, 1 out]
            n166 = Concatenate Strings(w382, "\r", w374) -> (w381:string)
            n167 = call "p9ctl.vi"("p9 action"=p9action_control."message", "message"=w381) -> ()  [unwired: 7 in, 3 out]
          }
          frame "itc box: read sweep table" {
            w403 = T33."table to rates"  # action
            # "read sweep table"
            n168 = call "itc Hg box controller -- wrapper -- A1.vi"("itc box action"=itc_503_box_-_control."read sweep table", "error in"=w401) -> ("error out"=w398:errorcluster, "Sweep Table"=w400:dbl[][])  [unwired: 7 in, 1 out]
            "Sweep Table" <- w400
            n169 = call "itc Hg box controller -- wrapper -- A1.vi"("itc box action"=itc_503_box_-_control."read state", "error in"=w398) -> ("error out"=w397:errorcluster, "itc box state OUT"=w395:T37)  [unwired: 7 in, 1 out]
            n170 = Unbundle By Name(w395) -> ("ITC set temperature"=w394:dbl)
            "current set temperature" <- w394
            n171 = call "sweep table staff.vi"("action"=w403, "Sweep Table"=w400, "set temperature IN"=w394) -> ("date string Array"=→"date string Array":string[], "Sweep Rates , min/K"=→"Sweep Rates , min/K":dbl[])  [unwired: 5 in, 2 out]
          }
          frame "itc box: set gas to" {
            n172 = call "itc Hg box controller -- wrapper -- A1.vi"("itc box action"=itc_503_box_-_control."set gas to", "error in"=w408, "input"="set gas % to") -> ("error out"=w407:errorcluster)  [unwired: 6 in, 2 out]
          }
          frame "itc box: set temperature to" {
            n173 = call "itc Hg box controller -- wrapper -- A1.vi"("itc box action"=itc_503_box_-_control."set temperature to", "error in"=w411, "input"="itc box: set temperature to: value") -> ("error out"=w410:errorcluster)  [unwired: 6 in, 2 out]
          }
          frame "itc box: set heater to" {
            n174 = call "itc Hg box controller -- wrapper -- A1.vi"("itc box action"=itc_503_box_-_control."set heater to", "error in"=w415, "input"="itc box: set heater to: value") -> ("error out"=w414:errorcluster)  [unwired: 6 in, 2 out]
          }
          frame "itc box: start/stop sweep" {
            n175 = local read "ITC panel"() -> (w420:T14)
            n176 = Unbundle By Name(w420) -> ("in sweep"=w421:bool)
            n177 = case shown="True" w421 {
              tunnel: [itc_503_box_-_control."start sweep" ("itc box action") itc_503_box_-_control."stop sweep" ("itc box action")] -> w417
              frame False {
                # "start sweep ..."
              }
              frame True {
                # "stop sweep ..."
              }
            }
            n178 = call "itc Hg box controller -- wrapper -- A1.vi"("itc box action"=w417, "error in"=w419) -> ("error out"=w418:errorcluster)  [unwired: 7 in, 2 out]
          }
          frame "itc box: write sweep table" {
            w424 = TRUE
            w438 = FALSE
            n179 = local write "Uploading ..."(w424) -> ()
            n180 = property on="Uploading ..." class="Bool (strict)"(error in=w437, "Visible"=w424) -> (error out=w429:errorcluster)  [unwired: 1 in, 1 out]
            n181 = case shown="True" "use" {
              tunnel: [w440 w445] -> w427
              tunnel: "new sweep table" -> [w440 w448]
              tunnel: "Rates , min/K" -> [w442 w449]
              tunnel: "set temperature" -> [w441 w450]
              frame False {
                n182 = call "sweep table staff.vi"("action"=T33."table to rates", "Sweep Table"=w440, "Sweep Rates , min/K IN"=w442, "set temperature IN"=w441) -> ("Sweep Rates , min/K"=w439:dbl[])  [unwired: 4 in, 3 out]
                n183 = local write "Rates , min/K"(w439) -> ()
              }
              frame True {
                n184 = call "sweep table staff.vi"("action"=T33."rates to table", "Sweep Table"=w448, "Sweep Rates , min/K IN"=w449, "set temperature IN"=w450) -> ("date string Array"=w444:string[], "Sweep Table"=w445:dbl[][], "Sweep Rates , min/K"=w446:dbl[])  [unwired: 4 in, 1 out]
                n185 = local write "new sweep table"(w445) -> ()
                n186 = local write "date string Array"(w444) -> ()
                n187 = local write "Sweep Rates , min/K"(w446) -> ()
              }
            }
            n188 = call "itc Hg box controller -- wrapper -- A1.vi"("itc box action"=itc_503_box_-_control."write sweep table", "error in"=w429, "Sweep Table In"=w427, "input"="set temperature") -> ("error out"=w425:errorcluster)  [unwired: 5 in, 2 out]
            n189 = local write "Uploading ..."(w438) -> ()
            n190 = property on="Uploading ..." class="Bool (strict)"(error in=w425, "Visible"=w438) -> (error out=w435:errorcluster)  [unwired: 1 in, 1 out]
            n191 = Generate User Event(user event=w436, event data cluster="itc box: read sweep table", error in=w435) -> (error out=w434:errorcluster)  [unwired: 1 in, 1 out]
          }
          frame "nothing", Default {
            w458 = FALSE  # quote specials
            # "intercept actions that do not match anything on the list"
            n192 = call "test for a regexp list.vi"("quote specials"=w458, "string"=w456, "regexps"=string[] ["itc\\ box:\\ set\\ gas\\ to\\ ([\\d\\.]+)", "itc\\ box:\\ set\\ temperature\\ to\\ ([\\d\\.]+)", "set:\\ new_sweep_table=(\\s*\\n)?((.*\\n?)+)", "set:\\ new_set_temperature=([\\d\\.]+)"]) -> ("match found"=w457:bool, "matching string index"=w453:i32, "matching regexp"=w455:string)  [unwired: 5 in, 1 out]
            n193 = case shown="True" w457 {
              tunnel: w456 -> [_ w462]
              tunnel: w455 -> [_ w460]
              tunnel: w453 -> [_ w461]
              tunnel: w451 -> [_ w459]
              frame False {
              }
              frame True {
                n194 = case shown="1" w461 {
                  tunnel: w462 -> [_ w466 w591 w720 w841]
                  tunnel: w460 -> [_ w465 w590 w721 w842]
                  tunnel: w459 -> [_ w464 w589 _ _]
                  frame -1, Default {
                  }
                  frame 1 {
                    n195 = xnode "Match Regular Expression"("input string"=w466, "regular expression"=w465) -> ("submatch 1"=w467:string)  [unwired: 4 in, 5 out]
                    n196 = flat-sequence {
                      tunnel: w467 -> [w472]
                      tunnel: w464 -> [w474]
                      tunnel: "itc box: set temperature to" ("action") -> [w473]
                      frame #0 {
                        w469 = 1.0  # lower
                        w470 = 330.0  # upper
                        n197 = Fract/Exp String To Number(string=w472) -> (number=w471:dbl)  [unwired: 3 in, 1 out]
                        n198 = call "Q -- check range.vi"("upper"=w470, "lower"=w469, "number"=w471) -> ("number in range"=w468:dbl)  [unwired: 4 in, 4 out]
                        n199 = local write "itc box: set temperature to: value"(w468) -> ()
                      }
                      frame #1 {
                        n200 = Generate User Event(user event=w474, event data cluster=w473) -> ()  [unwired: 2 in, 2 out]
                      }
                    }
                  }
                  frame 0 {
                    n201 = xnode "Match Regular Expression"("input string"=w591, "regular expression"=w590) -> ("submatch 1"=w592:string)  [unwired: 4 in, 5 out]
                    n202 = flat-sequence {
                      tunnel: w592 -> [w597]
                      tunnel: w589 -> [w599]
                      tunnel: "itc box: set gas to" ("action") -> [w598]
                      frame #0 {
                        w595 = 0.1  # lower
                        w596 = 99.0  # upper
                        n203 = Fract/Exp String To Number(string=w597) -> (number=w594:dbl)  [unwired: 3 in, 1 out]
                        n204 = call "Q -- check range.vi"("upper"=w596, "lower"=w595, "number"=w594) -> ("number in range"=w593:dbl)  [unwired: 4 in, 4 out]
                        n205 = local write "set gas % to"(w593) -> ()
                      }
                      frame #1 {
                        n206 = Generate User Event(user event=w599, event data cluster=w598) -> ()  [unwired: 2 in, 2 out]
                      }
                    }
                  }
                  frame 2 {
                    w714 = 0
                    (unwired) "\t"
                    n207 = local read "new sweep table"() -> (w716:dbl[][])
                    n208 = xnode "Match Regular Expression"("input string"=w720, "regular expression"=w721) -> ("submatch 2"=w718:string)  [unwired: 4 in, 6 out]
                    n209 = Spreadsheet String To Array(delimiter (Tab)=string[] [" ", "\t"], format string="%f " ("delimiter (Tab)"), spreadsheet string=w718) -> (array=w715:dbl[][])  [unwired: 1 in]
                    n210 = Replace Array Subset(array=w716, new element=w715, index (row)=w714, index (col)=w714) -> (w713:dbl[][])
                    n211 = local write "new sweep table"(w713) -> ()
                  }
                  frame 3 {
                    w837 = 330.0  # upper
                    w838 = 0.0  # lower
                    (unwired) "\t"
                    n212 = xnode "Match Regular Expression"("input string"=w841, "regular expression"=w842) -> ("submatch 1"=w840:string)  [unwired: 4 in, 5 out]
                    n213 = Fract/Exp String To Number(string=w840) -> (number=w839:dbl)  [unwired: 3 in, 1 out]
                    n214 = call "Q -- check range.vi"("upper"=w837, "lower"=w838, "number"=w839) -> ("number in range"=w836:dbl)  [unwired: 4 in, 4 out]
                    n215 = local write "set temperature"(w836) -> ()
                  }
                }
              }
            }
          }
          frame "overheat: check" {
            n216 = Unbundle By Name(w960) -> ("nonzero temperature"=w959:dbl)
            n217 = Not(x="Overheat !!") -> (.not. x?=w964:bool)
            n218 = Greater Or Equal?(x=w959, y="Over heat Temperature") -> (x >= y?=w963:bool)
            n219 = Compound Arithmetic op=AND("Overheat protection", w964, w963) -> (w962:bool)
            n220 = case shown="True" w962 {
              tunnel: [FALSE ("Boolean") TRUE ("Boolean")] -> w967
              tunnel: w958 -> [_ w969]
              tunnel: string[] ["gas flow: off", "rus loop: off", "itc box: off", "tabs: disable"] -> [_ w970]
              frame False {
                (unwired) TRUE ("Control Gas flow ?")
              }
              frame True {
                n221 = for {
                  tunnel: w969 -> [w973]
                  tunnel: w970 -> [w972] mode=indexing
                  n222 = Generate User Event(user event=w973, event data cluster=w972) -> ()  [unwired: 2 in, 2 out]
                }
              }
            }
            n223 = local write "Overheat !!"(w967) -> ()
          }
          frame "overheat: init" {
            n224 = call "sweep init checklist.vi"("action"=w975) -> ()  [unwired: 10 in, 1 out]
            n225 = local write "Overheat protection"(w976) -> ()
            n226 = local write "Overheat !!"(w976) -> ()
          }
          frame "rus loop: off" {
            n227 = local write "RUS loop"(w978) -> ()
          }
          frame "rus loop: on" {
            n228 = local write "RUS loop"(w980) -> ()
          }
          frame "save log: check" {
            n229 = local read "save log"() -> (w986:T23)
            n230 = call "save ITC log.vi"("action"=enum16{"init", "check"}."check", "file path"=w981, "temperature boxes"=w984, "seconds"=w985, "save log"=w986) -> ("saving log to"=w988:string, "save log out"=w987:T23)  [unwired: 5 in]
            n231 = local write "saving log to"(w988) -> ()
            n232 = local write "save log"(w987) -> ()
          }
          frame "save log: init" {
            n233 = call "sweep init checklist.vi"("action"=w992) -> ()  [unwired: 10 in, 1 out]
            n234 = call "save ITC log.vi"("action"=enum16{"init", "check"}."init", "seconds"=w990) -> ()  [unwired: 8 in, 2 out]
          }
          frame "stability log: write" {
            n235 = case shown="True" FALSE {
              tunnel: w996 -> [_ w999]
              tunnel: w994 -> [_ w998]
              frame False {
              }
              frame True {
                (unwired) "Stability_" ("current sweep file name")
                n236 = local read "file name prefix"() -> (w997:string)
                n237 = call "RUS Sweep -- write line to log file.vi"("temperature boxes"=w999, "base path"=w998, "current sweep file name"=w997, "base name"="Stability_") -> ("writing to"=→"writing log to":string, "log line"=→"log line":string)  [unwired: 5 in, 1 out]
              }
            }
          }
          frame "itc 503 controller: init" {
            # "this is supposed to be guaranteed to be the first (in time) call to ... wrapper ... vi. \nso it is enough to set protocol here only"
            n238 = call "sweep init checklist.vi"("action"=w1008) -> ()  [unwired: 10 in, 1 out]
            n239 = call "ctl -- name dispatcher.vi"("sweep folder path"=w1006, "ctl name dispatch"=ctl_--_name_dispatcher_--_action."errors" ("ctl kind")) -> ("file path"=w1005:path)  [unwired: 7 in, 2 out]
            n240 = case shown="\"do not use oxford ITC\"" w1004 {
              tunnel: [itc_503_box_-_control."enable" ("itc box action") itc_503_box_-_control."disable" ("itc box action")] -> w1012
              frame "use oxford ITC", Default {
              }
              frame "do not use oxford ITC" {
              }
            }
            n241 = Unbundle By Name("temperature boxes") -> ("ITC503 Address"=w1015:refnum<visa-resource-name>)
            n242 = call "itc Hg box controller -- wrapper -- A1.vi"("itc box protocol selector"="itc box protocol selector", "itc box action"=w1012, "error in"=w1010) -> ("error out"=w1014:errorcluster)  [unwired: 6 in, 2 out]
            n243 = call "itc Hg box controller -- wrapper -- A1.vi"("itc box protocol selector"="itc box protocol selector", "Log File Path"=w1005, "itc box action"=itc_503_box_-_control."init", "error in"=w1014, "VISA resource name"=w1015) -> ("error out"=w1009:errorcluster)  [unwired: 4 in, 2 out]
          }
          frame "itc 503 controller: check" {
            (unwired) u32 1  # plot every # sec
            w1030 = 60.0  # plot last (min)
            (unwired) u32 1  # aggregate every # sec
            w1029 = 10.0  # history length (min)
            n244 = control-ref of="ITC panel"() -> (w1018:refnum<vi>)
            n245 = call "ITC503 -- scan ITC LTC state -- Pgg1.vi"("error logfile path"=w1019, "disable interaction with itc"=w1020, "error in"=w1022, "state IN"=w1025) -> ("error out"=w1021:errorcluster, "itc box state OUT"=w1034:T37, "state OUT"=w1033:T21)  [unwired: 5 in]
            n246 = call "itc ltc - aggregate.vi"("aggregate every # sec"=w1023, "history length (min)"=w1029, "temperature boxes"=w1033) -> ("temperature indicator panel"=w1028:T19)  [unwired: 8 in]
            n247 = call "ITC panel controller -- Pgg1.vi"("itc box state IN"=w1034, "action"=T34."parse", "ITC panel IN"=w1018) -> ()  [unwired: 9 in]
            n248 = control-ref of="Plot: temperature"() -> (w1026:refnum<vi>)
            n249 = control-ref of="Plot: heater/gas"() -> (w1027:refnum<vi>)
            n250 = local write "temperature boxes"(w1033) -> ()
            n251 = local write "temperature indicator panel"(w1028) -> ()
            n252 = call "itc ltc plots.vi"("Plot: heater/gas"=w1027, "aggregate every # sec"=w1023, "Plot: temperature"=w1026, "plot length (min)"=w1030, "plot?"="plot?", "temperature indicator panel"=w1028, "time (sec)"=w1024) -> ()  [unwired: 5 in]
          }
          frame "sweep table: init" {
            w1038 = FALSE
            n253 = property on="Uploading ..." class="Bool (strict)"("Visible"=w1038) -> ()  [unwired: 2 in, 2 out]
            n254 = call "sweep init checklist.vi"("action"=w1036) -> ()  [unwired: 10 in, 1 out]
            "Uploading ..." <- w1038
            "saving sweep table to" <- "" ("saving sweep table to")
          }
          frame "sweep table: check" {
          }
          frame "tabs: check" {
          }
          frame "tabs: disable" {
            n255 = Select(t=T35."Disabled and Grayed Out" ("Disabled"), s=TRUE, f=T35."Enabled" ("Disabled")) -> (s? t:f=w1043:T35)
            n256 = property on="Tab: ITC controls" class="TabCtl (strict)"("DisabledEnum"=w1043) -> ()  [unwired: 2 in, 2 out]
          }
          frame "tabs: enable" {
            n257 = Select(t=T35."Disabled and Grayed Out" ("Disabled"), s=FALSE, f=T35."Enabled" ("Disabled")) -> (s? t:f=w1048:T35)
            n258 = property on="Tab: ITC controls" class="TabCtl (strict)"("DisabledEnum"=w1048) -> ()  [unwired: 2 in, 2 out]
          }
          frame "tabs: init" {
            n259 = call "sweep init checklist.vi"("action"=w1055) -> ()  [unwired: 10 in, 1 out]
            n260 = Select(t=T35."Disabled and Grayed Out" ("Disabled"), s=FALSE, f=T35."Enabled" ("Disabled")) -> (s? t:f=w1052:T35)
            n261 = property on="Tab: ITC controls" class="TabCtl (strict)"("DisabledEnum"=w1052) -> ()  [unwired: 2 in, 2 out]
          }
          frame "set temperature loop: init" {
            n262 = call "sweep init checklist.vi"("action"=w1058) -> ()  [unwired: 10 in, 1 out]
          }
          frame "set temperature loop: check" {
            n263 = call "sweep init checklist.vi"("action"=w1066) -> ()  [unwired: 10 in, 1 out]
            n264 = Unbundle By Name("Set Temperature PID") -> ("set temperature?"=w1061:bool)
            n265 = case shown="True" w1061 {
              tunnel: w1063 -> [_ w1084]
              tunnel: w1065 -> [w1067 w1082]
              tunnel: [w1067 w1081] -> w1064
              tunnel: w1062 -> [_ w1078]
              tunnel: "Set Temperature PID" -> [_ w1080]
              tunnel: w1059 -> [_ w1070]
              frame False {
              }
              frame True {
                n266 = Bundle By Name(cluster=w1080, "interval(sec)"=w1078) -> (w1079:T13)
                n267 = Unbundle By Name(w1070) -> ("LTC21 Address"=w1069:refnum<visa-resource-name>, "Neocera sensor"=w1068:i32)
                n268 = call "set temperature SINEWAVE - V1.vi"("sweep folder path"=w1084, "Set Temperature PID"=w1079) -> ("next set temperature"=w1083:dbl, "Set Temperature PID OUT"=w1072:T13)  [unwired: 6 in, 2 out]
                n269 = Unbundle By Name(w1072) -> ("Time(min)"=w1076:dbl, "Temperature(K)"=w1075:dbl, "OK?"=w1074:bool, "interval(sec)"=w1073:dbl)
                n270 = case shown="\"set T -> LTC (neocera)\"" "set Temperature target" {
                  tunnel: w1083 -> [w1091 w1095]
                  tunnel: w1082 -> [w1088 w1093]
                  tunnel: [w1087 w1092] -> w1081
                  tunnel: w1069 -> [w1090 _]
                  tunnel: w1068 -> [w1085 _]
                  frame "set T -> LTC (neocera)" {
                    n271 = call "Neocera21 Set T.vi"("Channel"=w1085, "Ramp rate, K/min"=0.03, "error in (no error)"=w1088, "Approach"=Set_Point_Aproach."Instant", "Set T"=w1091, "VISA Resource Name"=w1090) -> ("error out"=w1087:errorcluster)  [unwired: 4 in, 1 out]
                  }
                  frame "set T -> ITC (oxford)", Default {
                    n272 = call "itc Hg box controller -- wrapper -- A1.vi"("itc box action"=itc_503_box_-_control."set temperature to", "error in"=w1093, "input"=w1095) -> ("error out"=w1092:errorcluster)  [unwired: 6 in, 2 out]
                  }
                }
                n273 = Bundle By Name(cluster=w1072, "Time(min)"=w1076, "Temperature(K)"=w1075, "OK?"=w1074, "interval(sec)"=w1073) -> (w1077:T13)
                n274 = local write "Set Temperature PID"(w1077) -> ()
              }
            }
          }
        }
      }
      event Value Change {
        w1097 = "itc box: start/stop sweep"  # event data
        n275 = event-data() -> ()  [unwired: 1 in, 6 out]
        n276 = Generate User Event(user event=w1096, event data cluster=w1097) -> ()  [unwired: 2 in, 2 out]
      }
      event Value Change {
        n277 = event-data() -> ()  [unwired: 1 in, 2 out]
        n278 = Unbundle By Name(w1104) -> ("nonzero temperature"=w1103:dbl)
        n279 = local read "Fast sweep settings"() -> (w1101:T6)
        n280 = call "file name prefix.vi"("Fast sweep settings"=w1101, "temperature"=w1103) -> ("minutes/sweep"=w1100:dbl, "kHz/second"=w1108:dbl, "file name prefix"=w1106:string)  [unwired: 6 in, 1 out]
        n281 = local write "sweep time  (min)"(w1100) -> ()
        n282 = Bundle By Name(cluster=w1107, "File Prefix"=w1106) -> (w1105:T7)
        n283 = Multiply(x=60.0, y=w1100) -> (x*y=→"sweep time (sec)":dbl)
        n284 = local write "kHz/second"(w1108) -> ()
        n285 = local write "Save data settings"(w1105) -> ()
      }
      event Value Change {
        w1109 = "gas flow: set gas to"  # event data
        n286 = event-data() -> ()  [unwired: 1 in, 6 out]
        n287 = Generate User Event(user event=w1110, event data cluster=w1109) -> ()  [unwired: 2 in, 2 out]
      }
      event Value Change {
        w1113 = "gas flow: force up"  # event data
        n288 = event-data() -> ()  [unwired: 1 in, 6 out]
        n289 = Generate User Event(user event=w1114, event data cluster=w1113) -> ()  [unwired: 2 in, 2 out]
      }
      event Value Change {
        w1117 = "gas flow: force down"  # event data
        n290 = event-data() -> ()  [unwired: 1 in, 6 out]
        n291 = Generate User Event(user event=w1116, event data cluster=w1117) -> ()  [unwired: 2 in, 2 out]
      }
      event Value Change {
        w1120 = "gas flow: stop up/down"  # event data
        n292 = event-data() -> ()  [unwired: 1 in, 6 out]
        n293 = Generate User Event(user event=w1119, event data cluster=w1120) -> ()  [unwired: 2 in, 2 out]
      }
      event Value Change {
        w1127 = T38."turn on"  # action
        w1128 = T38."turn off"  # action
        n294 = event-data() -> ("NewVal"=w1125:bool)  [unwired: 1 in]
        n295 = Select(t=w1127, s=w1125, f=w1128) -> ()  [unwired: 1 out]
        n296 = Select(t="gas flow: on" ("event data"), s=w1125, f="gas flow: off" ("event data")) -> (s? t:f=w1122:string)
        n297 = Generate User Event(user event=w1126, event data cluster=w1122) -> ()  [unwired: 2 in, 2 out]
      }
      event Value Change {
        n298 = event-data() -> ()  [unwired: 1 in, 6 out]
        n299 = call "gas flow controller -- Pgg3.vi"("action"=gas_flow_controller_action."update parameters") -> ()  [unwired: 10 in, 1 out]
      }
      event Value Change {
        w1132 = "alarm clock: start"  # event data
        n300 = event-data() -> ()  [unwired: 1 in, 2 out]
        n301 = Generate User Event(user event=w1133, event data cluster=w1132) -> ()  [unwired: 2 in, 2 out]
      }
      event Value Change {
        w1135 = "alarm clock: stop"  # event data
        n302 = event-data() -> ()  [unwired: 1 in, 2 out]
        n303 = Generate User Event(user event=w1136, event data cluster=w1135) -> ()  [unwired: 2 in, 2 out]
      }
    }
    n304 = call "BypassAndLogErrors -- V2.vi"("Bypass Errors"=w163, "error in (no error)"=w162, "Log File Path"=w159) -> ("error out"=w161:errorcluster)  [unwired: 8 in]
  }
  n305 = local write "seconds"(w1) -> ()
  n306 = while {
    tunnel: w8 -> [w1151]
    shift-right: [w1142] -> _
    shift-left: w5 -> [w1141]
    shift-right: [w1138] -> _
    shift-left: w3 -> [w1138]
    tunnel: w1 -> [_]
    i -> [w1146]
    stop <- FALSE ("Boolean") stop-if-true
    w1143 = u32 1000 ("milliseconds per cycle")
    w1149 = TRUE  # run dispatch loop
    w1145 = u32 6153 ("milliseconds per cycle")
    # "dispatch loop"
    n307 = Tick Count (ms)() -> (millisecond timer value=w1140:u32)
    n308 = Equal To 0?(x=w1146) -> (x = 0?=w1154:bool)
    n309 = Subtract(x=w1140, y=w1138) -> (x-y=w1139:u32)
    n310 = Divide(x=w1139, y=w1143) -> (x/y=w1137:dbl)
    "seconds" <- w1137
    n311 = case shown="True" w1154 {
      tunnel: w1141 -> [w1166 w1169]
      tunnel: [w1166 w1167] -> w1152
      tunnel: w1137 -> [_ _]
      frame False {
      }
      frame True {
        w1168 = "all: init" ("event data")
        n312 = Generate User Event(user event=w1169, event data cluster=w1168) -> (user event out=w1167:refnum<user-event>)  [unwired: 2 in, 1 out]
        n313 = call "sweep init checklist.vi"("action"=w1168) -> ()  [unwired: 10 in, 1 out]
      }
    }
    n314 = Divide(x=w1137, y=60) -> (x/y=→"minutes":dbl)
    n315 = Wait (ms)(milliseconds to wait=w1145) -> ()  [unwired: 1 out]
    n316 = Divide(x=w1145, y=w1143) -> (x/y=→"seconds per cycle":dbl)
    n317 = call "sweep init checklist.vi"("action"="test" ("event data")) -> ("result"=w1148:bool)  [unwired: 10 in]
    n318 = And(x=w1149, y=w1148) -> (x .and. y?=w1147:bool)
    n319 = case shown="True" w1147 {
      tunnel: w1152 -> [w1157 w1159]
      tunnel: w1151 -> [_ w1160]
      tunnel: [w1157 w1158] -> w1142
      frame False {
      }
      frame True {
        n320 = for {
          tunnel: w1160 -> [w1165] mode=indexing
          shift-right: [w1162] -> w1158
          shift-left: w1159 -> [w1161]
          n321 = Concatenate Strings(w1165, " check" ("event data")) -> (w1163:string)
          n322 = Generate User Event(user event=w1161, event data cluster=w1163) -> (user event out=w1162:refnum<user-event>)  [unwired: 2 in, 1 out]
        }
      }
    }
    "milliseconds per cycle" <- w1145
  }
  n323 = disable-structure shown="Disabled" {
    disable-tunnel: _ -> [w1170 _]
    frame Disabled {
      n324 = for {
        tunnel: w1170 -> [w1176]
        tunnel: i32[] [3, 4, 5, 6] -> [w1172] mode=indexing
        # "pid contro page"
        n325 = property on="Tab: everything" class="TabCtl (strict)"() -> ("Pages"=w1178:refnum<vi>[])  [unwired: 2 in, 2 out]
        n326 = Select(t=T39."Page Disabled & Grayed" ("Page Enabled State"), s=w1176, f=T39."Page Enabled" ("Page Enabled State")) -> (s? t:f=w1173:T39)
        n327 = Index Array(array=w1178, index=w1172) -> (element=w1177:refnum<vi>)
        n328 = property on="Property Node" class="Page"(reference=w1177, "PageEnb"=w1173) -> ()  [unwired: 1 in, 2 out]
      }
    }
    frame Enabled {
    }
  }
